vi "Parameter Analyzer.vi"(0 "Function":T3, 1 "Acquisition Mode":T7, 2 "User Integration Time":T9={"Integration Time"=0, "Short Integration Time (s)"=0.0, "Long Integration Time (s)"=0.0, "Wait Time Parameter"=1.0} caption="Sweeping Time Parameters" {"Long Integration Time (s)" scale=0.02..2.0; "Short Integration Time (s)" scale=8e-05..0.00192; "Integration Time" items=["Short", "Long"]; "Wait Time Parameter" format="%.1f"}, 3 "Status Polling Time (ms)":u32=1000, 4 "VISA Session":refnum<visa-resource-name>="GPIB0::27::INSTR", 5 "Comment":string="Test VI", 6 "HP4155C Refnums":T5, 7 "Error in":errorcluster, 8 "SMU 1 - Sweeping":T8={"Start / Offset"=0.0, "Stop / Ratio"=1.0, "Step \n(linear only)"=0.01, "Compliance"=0.1, "Power \nCompliance"=0.0, "Mode"=0, "Function"=0, "Sweep Mode"=FALSE} caption="SMU 1" {"Function" items=["Disabled", "Var 1", "Var 2", "Var 1'", "Constant"]; "Mode" items=["V", "I", "V pulse", "I  pulse", "Common"]; "Power \nCompliance" format="%^.2e"; "Compliance" format="%^.2e"; "Step \n(linear only)" format="%^.4e"; "Stop / Ratio" format="%^.4e"; "Start / Offset" format="%^.4e"}, 9 "SMU1 - Sampling":T12={"Source"=10.0, "Compliance"=1e-05, "Mode"=0, "Function"=FALSE} caption="SMU 1" {"Mode" items=["V", "I", "Common"]; "Compliance" format="%^.2e"; "Source" format="%^.3e"}, 10 "SMU 2 - Sweeping":T8={"Start / Offset"=0.0, "Stop / Ratio"=1.0, "Step \n(linear only)"=0.01, "Compliance"=0.1, "Power \nCompliance"=0.0, "Mode"=0, "Function"=0, "Sweep Mode"=FALSE} caption="SMU 2" {"Function" items=["Disabled", "Var 1", "Var 2", "Var 1'", "Constant"]; "Mode" items=["V", "I", "V pulse", "I  pulse", "Common"]; "Power \nCompliance" format="%^.2e"; "Compliance" format="%^.2e"; "Step \n(linear only)" format="%^.4e"; "Stop / Ratio" format="%^.4e"; "Start / Offset" format="%^.4e"}, 11 "SMU2 - Sampling":T12={"Source"=10.0, "Compliance"=1e-05, "Mode"=0, "Function"=FALSE} caption="SMU 2" {"Mode" items=["V", "I", "Common"]; "Compliance" format="%^.2e"; "Source" format="%^.3e"}, 12 "SMU 3 - Sweeping":T8={"Start / Offset"=0.0, "Stop / Ratio"=1.0, "Step \n(linear only)"=0.01, "Compliance"=0.1, "Power \nCompliance"=0.0, "Mode"=0, "Function"=0, "Sweep Mode"=FALSE} caption="SMU 3" {"Function" items=["Disabled", "Var 1", "Var 2", "Var 1'", "Constant"]; "Mode" items=["V", "I", "V pulse", "I  pulse", "Common"]; "Power \nCompliance" format="%^.2e"; "Compliance" format="%^.2e"; "Step \n(linear only)" format="%^.4e"; "Stop / Ratio" format="%^.4e"; "Start / Offset" format="%^.4e"}, 13 "SMU3 - Sampling":T12={"Source"=10.0, "Compliance"=1e-05, "Mode"=0, "Function"=FALSE} caption="SMU 3" {"Mode" items=["V", "I", "Common"]; "Compliance" format="%^.2e"; "Source" format="%^.3e"}, 14 "SMU 4 - Sweeping":T8={"Start / Offset"=0.0, "Stop / Ratio"=1.0, "Step \n(linear only)"=0.01, "Compliance"=0.1, "Power \nCompliance"=0.0, "Mode"=0, "Function"=0, "Sweep Mode"=FALSE} caption="SMU 4" {"Function" items=["Disabled", "Var 1", "Var 2", "Var 1'", "Constant"]; "Mode" items=["V", "I", "V pulse", "I  pulse", "Common"]; "Power \nCompliance" format="%^.2e"; "Compliance" format="%^.2e"; "Step \n(linear only)" format="%^.4e"; "Stop / Ratio" format="%^.4e"; "Start / Offset" format="%^.4e"}, 15 "SMU4 - Sampling":T12={"Source"=10.0, "Compliance"=1e-05, "Mode"=0, "Function"=FALSE} caption="SMU 4" {"Mode" items=["V", "I", "Common"]; "Compliance" format="%^.2e"; "Source" format="%^.3e"}, 16 "Sweep Spacing":T11 items=["linear", "log 10", "log 25", "log 50"], 17 "Sampling Time Parameters":T13={"Initial Interval (s)"=0.1, "Number of Samples"=60, "Total Sampling Time (s)"=10.0, "Hold Time (s)"=0.0, "Sampling Mode"=0, "Sampling Time"=0} {"Sampling Time" items=["Auto (linear only)", "No Limit", "Set Limit"]; "Sampling Mode" items=["Linear", "Log10", "Log25", "Log50", "Thinned Out"]; "Hold Time (s)" format="%.4f"; "Total Sampling Time (s)" format="%.1f"; "Initial Interval (s)" format="%^.3e"}, 18 "Range":T10 items=["auto", "fixed", "limited"], 19 "Stop Condition":T14={"Enable Delay (s)"=0.0, "Name"="", "Threshold"=0.0, "num. of events"=1, "Event"=0, "Stop Condition Enable"=FALSE} {"Event" items=["Value > Threshold", "Value < Threshold", "| Value | > | Threshold |", "| Value | < | Threshold |"]; "Threshold" format="%^.2e"; "Enable Delay (s)" format="%.1f"}, 20 "Parameter Analyzer Notifiers":T4) -> (22 "Electrical Measurement":T15, 27 "error out":errorcluster)   [LabVIEW 2014]
uses:
  Parameter Analyzer Integration Parameters.ctl
  Electrical Data.ctl
  Parameter Analyzer SMU Sweeping.ctl
  Parameter Analyzer Sweep Spacing.ctl
  Parameter Analyzer Mode Selector.ctl
  Parameter Analyzer Sampling Parameters.ctl
  Parameter Analyzer Stop Sampling Conditions.ctl
  Parameter Analyzer SMU Sampling.ctl
  Parameter Analyzer Refnums.ctl
  Measurements/Plot Data/Electrical Data Plot Refnums.ctl
  Parameter Analyzer Notifiers.ctl
  Parameter Analyzer Functions.ctl
  Parameter Analyzer SMU Range.ctl
  support/Instrument Status.ctl
  support/Instrument Status State.ctl
  <instrlib>/Agilent 415X Series/Agilent 415X Series.lvlib
panel:
  in  "Electrical Measurement":T1(tab)
  out "Current Plot 2":cluster{"Time":dbl[], "SMU4":dbl[]}[](graph)=[{"Time"=[0.0, 0.30000000000000004, 0.6000000000000001, 0.9, 1.2000000000000002, 1.5, 1.8, 2.1, 2.4000000000000004, 2.7, 3.0, 3.3000000000000003, 3.6, 3.9000000000000004, 4.2, 4.5, 4.800000000000001, 5.1000000000000005, 5.4, 5.7, 6.0, 6.300000000000001, 6.6000000000000005, 6.9, 7.2, 7.5, 7.800000000000001, 8.1, 8.4, 8.700000000000001, 9.0, 9.3, 9.600000000000001, 9.9, 10.200000000000001, 10.5, 10.8, 11.100000000000001, 11.4, 11.700000000000001, 12.0, 12.3, 12.600000000000001, 12.9, 13.200000000000001, 13.5, 13.8, 14.100000000000001, 14.4, 14.700000000000001, 15.0, 15.3, 15.600000000000001, 15.9, 16.2, 16.5, 16.8, 17.1, 17.400000000000002, 17.7], "SMU4"=[9.99995e-06, 9.99995e-06, 9.99995e-06, 9.99997e-06, 9.99997e-06, 9.99997e-06, 9.99997e-06, 9.999980000000001e-06, 9.99997e-06, 9.999980000000001e-06, 9.99997e-06, 9.999980000000001e-06, 9.99997e-06, 9.99997e-06, 9.99997e-06, 9.99996e-06, 9.99996e-06, 9.99996e-06, 9.99996e-06, 9.99997e-06, 9.99997e-06, 9.999980000000001e-06, 9.99997e-06, 9.99997e-06, 9.99997e-06, 9.99997e-06, 9.99997e-06, 9.999980000000001e-06, 9.999980000000001e-06, 9.99996e-06, 9.99997e-06, 9.99996e-06, 9.99997e-06, 9.99997e-06, 9.99997e-06, 9.99997e-06, 9.999980000000001e-06, 9.99997e-06, 9.999980000000001e-06, 9.999980000000001e-06, 9.99997e-06, 9.99997e-06, 9.99997e-06, 9.99996e-06, 9.99996e-06, 9.99997e-06, 9.99997e-06, 9.99996e-06, 9.99996e-06, 9.99997e-06, 9.99997e-06, 9.99997e-06, 9.99997e-06, 9.99997e-06, 9.99996e-06, 9.99997e-06, 9.99997e-06, 9.99997e-06, 9.99997e-06, 9.99996e-06]}, {"Time"=[0.0, 0.30000000000000004, 0.6000000000000001, 0.9, 1.2000000000000002, 1.5, 1.8, 2.1, 2.4000000000000004, 2.7, 3.0, 3.3000000000000003, 3.6, 3.9000000000000004, 4.2, 4.5, 4.800000000000001, 5.1000000000000005, 5.4, 5.7, 6.0, 6.300000000000001, 6.6000000000000005, 6.9, 7.2, 7.5, 7.800000000000001, 8.1, 8.4, 8.700000000000001, 9.0, 9.3, 9.600000000000001, 9.9, 10.200000000000001, 10.5, 10.8, 11.100000000000001, 11.4, 11.700000000000001, 12.0, 12.3, 12.600000000000001, 12.9, 13.200000000000001, 13.5, 13.8, 14.100000000000001, 14.4, 14.700000000000001, 15.0, 15.3, 15.600000000000001, 15.9, 16.2, 16.5, 16.8, 17.1, 17.400000000000002, 17.7], "SMU4"=[-1.00004e-05, -1.000039e-05, -1.000039e-05, -1.0000409999999999e-05, -1.000039e-05, -1.000039e-05, -1.00004e-05, -1.000043e-05, -1.000042e-05, -1.0000409999999999e-05, -1.000039e-05, -1.000039e-05, -1.0000409999999999e-05, -1.00004e-05, -1.000038e-05, -1.000038e-05, -1.000039e-05, -1.000037e-05, -1.000038e-05, -1.000039e-05, -1.000039e-05, -1.000039e-05, -1.000039e-05, -1.000039e-05, -1.00004e-05, -1.000037e-05, -1.000038e-05, -1.000039e-05, -1.00004e-05, -1.00004e-05, -1.00004e-05, -1.000037e-05, -1.000037e-05, -1.000037e-05, -1.000036e-05, -1.000039e-05, -1.000038e-05, -1.000037e-05, -1.000036e-05, -1.000037e-05, -1.000038e-05, -1.000037e-05, -1.000038e-05, -1.000036e-05, -1.000037e-05, -1.000037e-05, -1.000037e-05, -1.000039e-05, -1.000038e-05, -1.000036e-05, -1.000037e-05, -1.000039e-05, -1.000036e-05, -1.000037e-05, -1.000038e-05, -1.00004e-05, -1.0000409999999999e-05, -1.000038e-05, -1.000038e-05, -1.00004e-05]}]
  out "Voltage Plot 2":cluster{"Time":dbl[], "SMU4":dbl[]}[](graph)=[{"Time"=[0.0, 0.30000000000000004, 0.6000000000000001, 0.9, 1.2000000000000002, 1.5, 1.8, 2.1, 2.4000000000000004, 2.7, 3.0, 3.3000000000000003, 3.6, 3.9000000000000004, 4.2, 4.5, 4.800000000000001, 5.1000000000000005, 5.4, 5.7, 6.0, 6.300000000000001, 6.6000000000000005, 6.9, 7.2, 7.5, 7.800000000000001, 8.1, 8.4, 8.700000000000001, 9.0, 9.3, 9.600000000000001, 9.9, 10.200000000000001, 10.5, 10.8, 11.100000000000001, 11.4, 11.700000000000001, 12.0, 12.3, 12.600000000000001, 12.9, 13.200000000000001, 13.5, 13.8, 14.100000000000001, 14.4, 14.700000000000001, 15.0, 15.3, 15.600000000000001, 15.9, 16.2, 16.5, 16.8, 17.1, 17.400000000000002, 17.7], "SMU4"=[9.99995e-06, 9.99995e-06, 9.99995e-06, 9.99997e-06, 9.99997e-06, 9.99997e-06, 9.99997e-06, 9.999980000000001e-06, 9.99997e-06, 9.999980000000001e-06, 9.99997e-06, 9.999980000000001e-06, 9.99997e-06, 9.99997e-06, 9.99997e-06, 9.99996e-06, 9.99996e-06, 9.99996e-06, 9.99996e-06, 9.99997e-06, 9.99997e-06, 9.999980000000001e-06, 9.99997e-06, 9.99997e-06, 9.99997e-06, 9.99997e-06, 9.99997e-06, 9.999980000000001e-06, 9.999980000000001e-06, 9.99996e-06, 9.99997e-06, 9.99996e-06, 9.99997e-06, 9.99997e-06, 9.99997e-06, 9.99997e-06, 9.999980000000001e-06, 9.99997e-06, 9.999980000000001e-06, 9.999980000000001e-06, 9.99997e-06, 9.99997e-06, 9.99997e-06, 9.99996e-06, 9.99996e-06, 9.99997e-06, 9.99997e-06, 9.99996e-06, 9.99996e-06, 9.99997e-06, 9.99997e-06, 9.99997e-06, 9.99997e-06, 9.99997e-06, 9.99996e-06, 9.99997e-06, 9.99997e-06, 9.99997e-06, 9.99997e-06, 9.99996e-06]}, {"Time"=[0.0, 0.30000000000000004, 0.6000000000000001, 0.9, 1.2000000000000002, 1.5, 1.8, 2.1, 2.4000000000000004, 2.7, 3.0, 3.3000000000000003, 3.6, 3.9000000000000004, 4.2, 4.5, 4.800000000000001, 5.1000000000000005, 5.4, 5.7, 6.0, 6.300000000000001, 6.6000000000000005, 6.9, 7.2, 7.5, 7.800000000000001, 8.1, 8.4, 8.700000000000001, 9.0, 9.3, 9.600000000000001, 9.9, 10.200000000000001, 10.5, 10.8, 11.100000000000001, 11.4, 11.700000000000001, 12.0, 12.3, 12.600000000000001, 12.9, 13.200000000000001, 13.5, 13.8, 14.100000000000001, 14.4, 14.700000000000001, 15.0, 15.3, 15.600000000000001, 15.9, 16.2, 16.5, 16.8, 17.1, 17.400000000000002, 17.7], "SMU4"=[-1.00004e-05, -1.000039e-05, -1.000039e-05, -1.0000409999999999e-05, -1.000039e-05, -1.000039e-05, -1.00004e-05, -1.000043e-05, -1.000042e-05, -1.0000409999999999e-05, -1.000039e-05, -1.000039e-05, -1.0000409999999999e-05, -1.00004e-05, -1.000038e-05, -1.000038e-05, -1.000039e-05, -1.000037e-05, -1.000038e-05, -1.000039e-05, -1.000039e-05, -1.000039e-05, -1.000039e-05, -1.000039e-05, -1.00004e-05, -1.000037e-05, -1.000038e-05, -1.000039e-05, -1.00004e-05, -1.00004e-05, -1.00004e-05, -1.000037e-05, -1.000037e-05, -1.000037e-05, -1.000036e-05, -1.000039e-05, -1.000038e-05, -1.000037e-05, -1.000036e-05, -1.000037e-05, -1.000038e-05, -1.000037e-05, -1.000038e-05, -1.000036e-05, -1.000037e-05, -1.000037e-05, -1.000037e-05, -1.000039e-05, -1.000038e-05, -1.000036e-05, -1.000037e-05, -1.000039e-05, -1.000036e-05, -1.000037e-05, -1.000038e-05, -1.00004e-05, -1.0000409999999999e-05, -1.000038e-05, -1.000038e-05, -1.00004e-05]}]
  out "Differential Resistance":cluster{"V3":dbl[], "I1":dbl[]}[](graph)
  out "Current Voltage Characteristic":cluster{"V3":dbl[], "I1":dbl[]}[](graph)
  out "Instrument Status":T2
  out "Error Messages":string
  out "Status":T16(ring)=enum."idle"
  out "HP Integration Time":T17={"Short Integration Time"=0.00192, "Medium Integration Time"=0.02, "Long Integration Time"=0.32} caption="Integration Time" {"Long Integration Time" format="%^.2e"; "Medium Integration Time" format="%^.2e"; "Short Integration Time" format="%^.2e"}
  # "LICENSED MATERIALS – PROPERTY OF IBM\nCopyright IBM Corp. 2016,\nALL RIGHTS RESERVED"
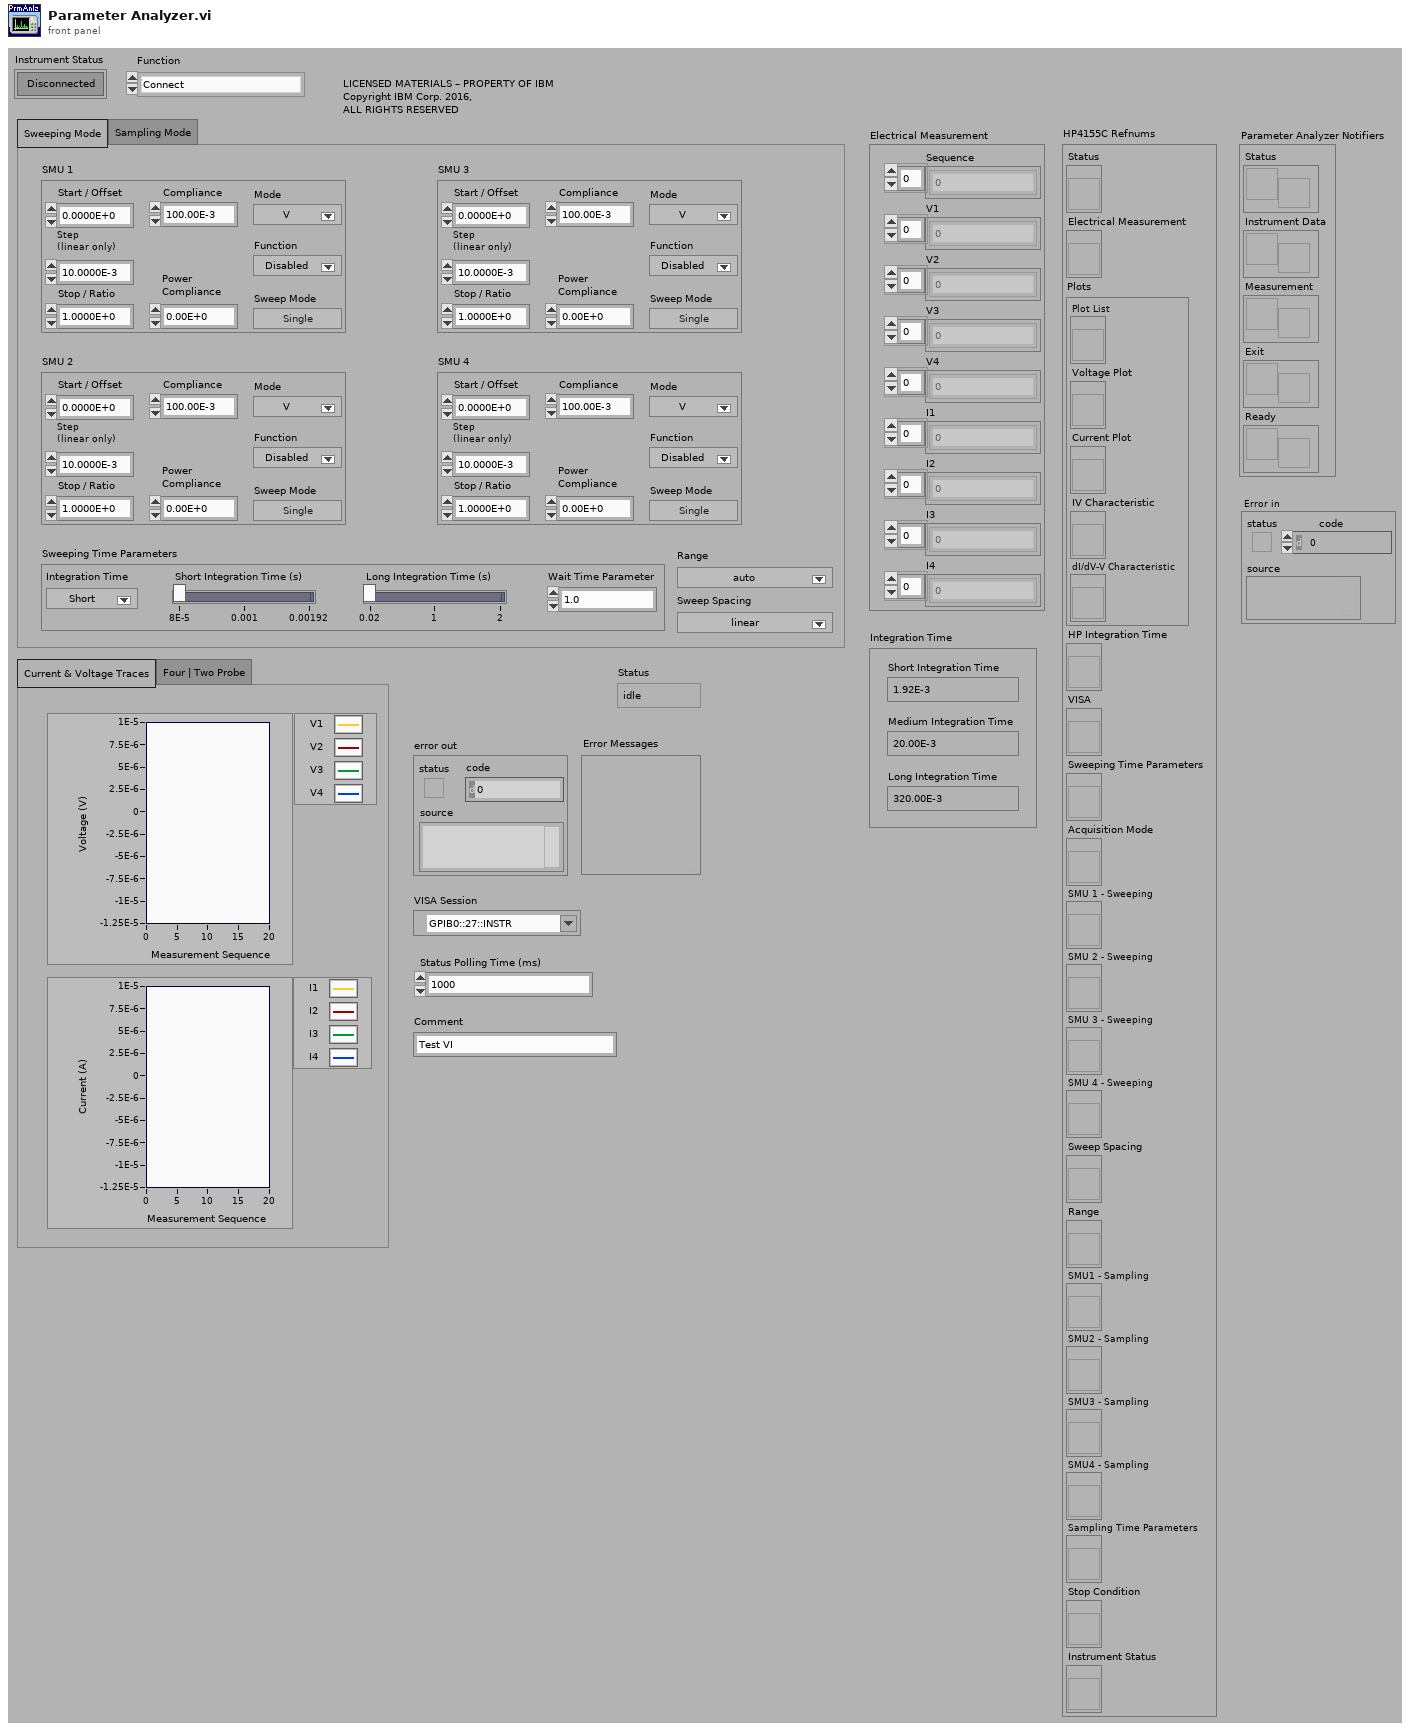
[diagram p1: front panel]
types:
  T1 = enum32{"Current & Voltage Traces", "Four | Two Probe"}
  T2 = typedef "Instrument Status.ctl" = bool
  T3 = typedef "Parameter Analyzer Functions.ctl" = enum16{"Connect", "Configure Sweeping", "Configure Sampling", "Configure Integration Time", "Measure", "Error Check", "Disconnect", "Update Refnums"}
  T4 = typedef "Parameter Analyzer Notifiers.ctl" = cluster{"Status":refnum<notifier>, "Instrument Data":refnum<notifier>, "Measurement":refnum<notifier>, "Exit":refnum<notifier>, "Ready":refnum<notifier>}
  T5 = typedef "Parameter Analyzer Refnums.ctl" = cluster{"Status":refnum<vi>, "Electrical Measurement":refnum<vi>, "Plots":T6, "HP Integration Time":refnum<vi>, "VISA":refnum<vi>, "Sweeping Time Parameters":refnum<vi>, "Acquisition Mode":refnum<vi>, "SMU 1 - Sweeping":refnum<vi>, "SMU 2 - Sweeping":refnum<vi>, "SMU 3 - Sweeping":refnum<vi>, "SMU 4 - Sweeping":refnum<vi>, "Sweep Spacing":refnum<vi>, "Range":refnum<vi>, "SMU1 - Sampling":refnum<vi>, "SMU2 - Sampling":refnum<vi>, "SMU3 - Sampling":refnum<vi>, "SMU4 - Sampling":refnum<vi>, "Sampling Time Parameters":refnum<vi>, "Stop Condition":refnum<vi>, "Instrument Status":refnum<vi>}
  T6 = typedef "Electrical Data Plot Refnums.ctl" = cluster{"Plot List":refnum<vi>, "Voltage Plot":refnum<vi>, "Current Plot":refnum<vi>, "IV Characteristic":refnum<vi>, "dI/dV-V Characteristic":refnum<vi>}
  T7 = typedef "Parameter Analyzer Mode Selector.ctl" = enum32{"Sweeping Mode", "Sampling Mode"}
  T8 = typedef "Parameter Analyzer SMU Sweeping.ctl" = cluster{"Start / Offset":dbl, "Stop / Ratio":dbl, "Step \n(linear only)":dbl, "Compliance":dbl, "Power \nCompliance":dbl, "Mode":u32, "Function":i32, "Sweep Mode":bool}
  T9 = typedef "Parameter Analyzer Integration Parameters.ctl" = cluster{"Integration Time":u32, "Short Integration Time (s)":dbl, "Long Integration Time (s)":dbl, "Wait Time Parameter":dbl}
  T10 = typedef "Parameter Analyzer SMU Range.ctl" = u16
  T11 = typedef "Parameter Analyzer Sweep Spacing.ctl" = u16
  T12 = typedef "Parameter Analyzer SMU Sampling.ctl" = cluster{"Source":dbl, "Compliance":dbl, "Mode":u32, "Function":bool}
  T13 = typedef "Parameter Analyzer Sampling Parameters.ctl" = cluster{"Initial Interval (s)":dbl, "Number of Samples":i32, "Total Sampling Time (s)":dbl, "Hold Time (s)":dbl, "Sampling Mode":i32, "Sampling Time":i32}
  T14 = typedef "Parameter Analyzer Stop Sampling Conditions.ctl" = cluster{"Enable Delay (s)":dbl, "Name":string, "Threshold":dbl, "num. of events":i32, "Event":i32, "Stop Condition Enable":bool}
  T15 = typedef "Electrical Data.ctl" = cluster{"Sequence":dbl[], "V1":dbl[], "V2":dbl[], "V3":dbl[], "V4":dbl[], "I1":dbl[], "I2":dbl[], "I3":dbl[], "I4":dbl[]}
  T16 = enum16{"unknown", "idle", "standby", "measurement", "stress force"}
  T17 = cluster{"Short Integration Time":dbl, "Medium Integration Time":dbl, "Long Integration Time":dbl}
  T18 = typedef "Instrument Status State.ctl" = enum16{"Unknown", "Idle", "Standby", "Configuring", "Measuring", "Moving", "Disconnected"}
  T19 = cluster{"unit (VMU1:0)":u16, "range (fixed:1)":u16, "SMU I range\n(1 nA:2)":u16, "SMU V range\n(2 V:0)":u16, "VMU range\n(2 V:1)":u16}[]
  T20 = cluster{"unit (VMU1:0)":u16, "range (fixed:1)":u16, "SMU I range\n(1 nA:2)":u16, "SMU V range\n(2 V:0)":u16, "VMU range\n(2 V:1)":u16}
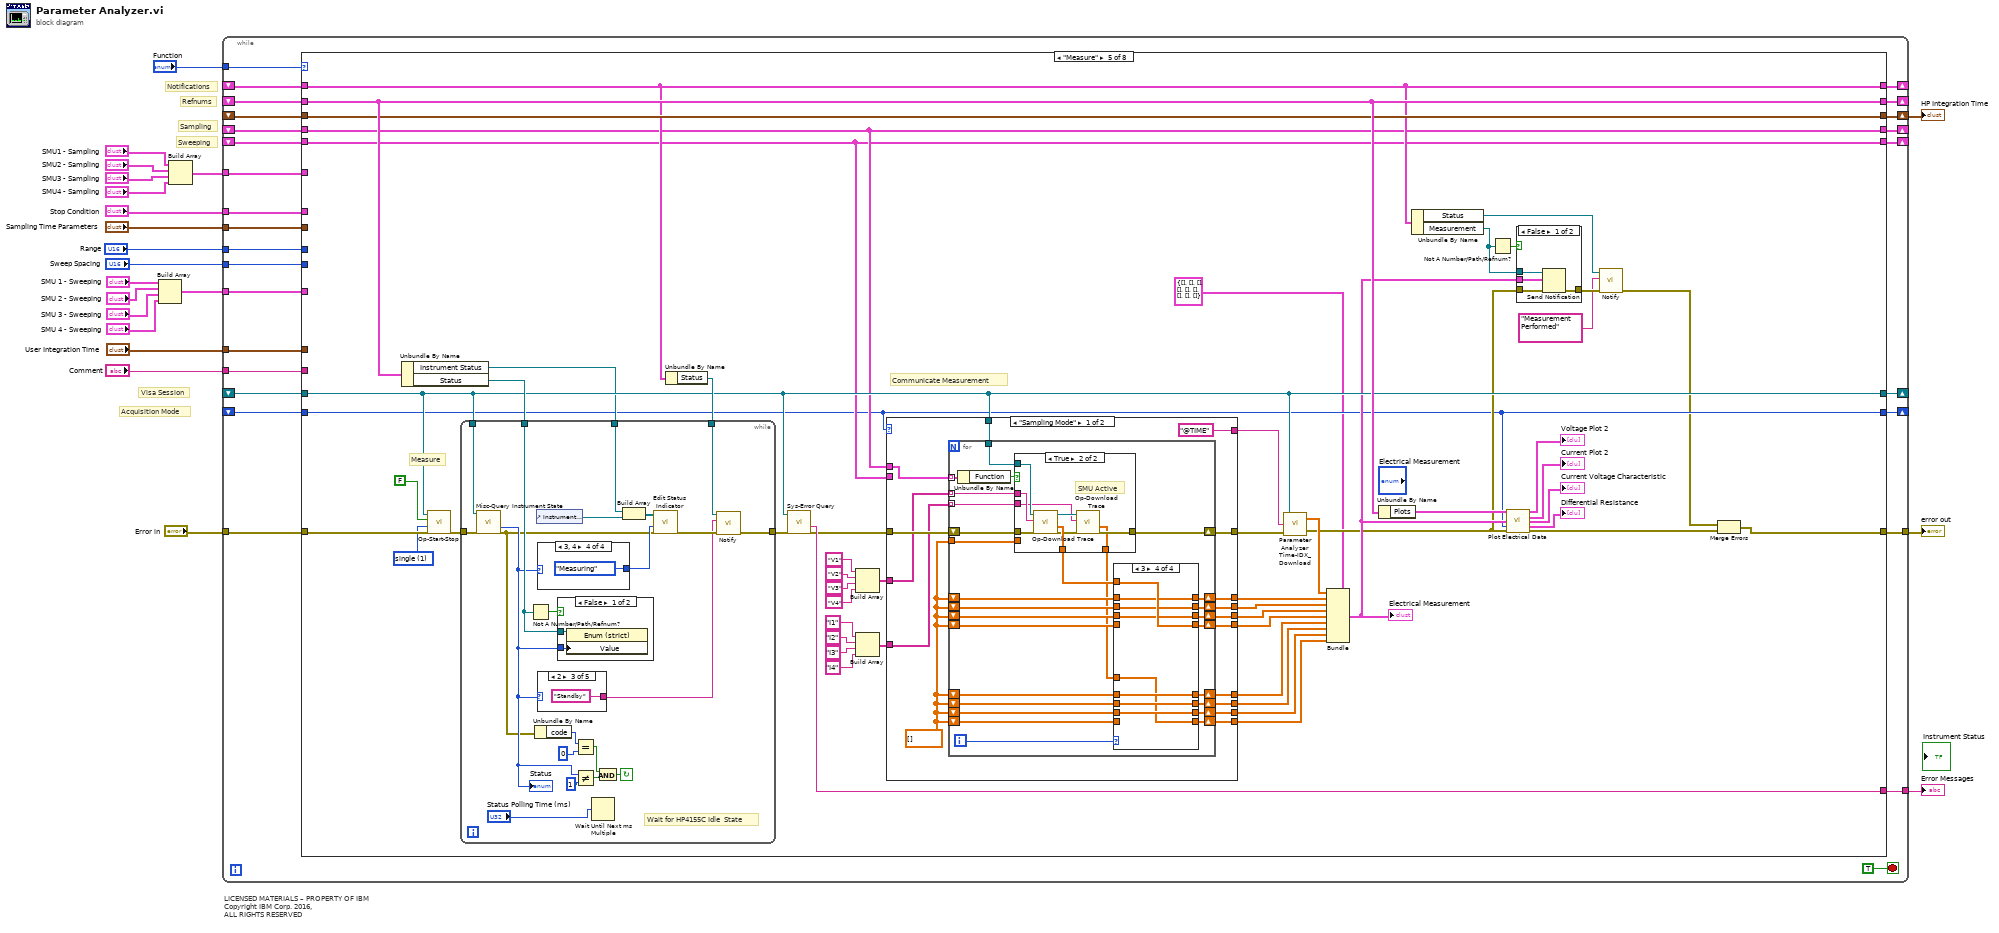
[diagram p0: block diagram]
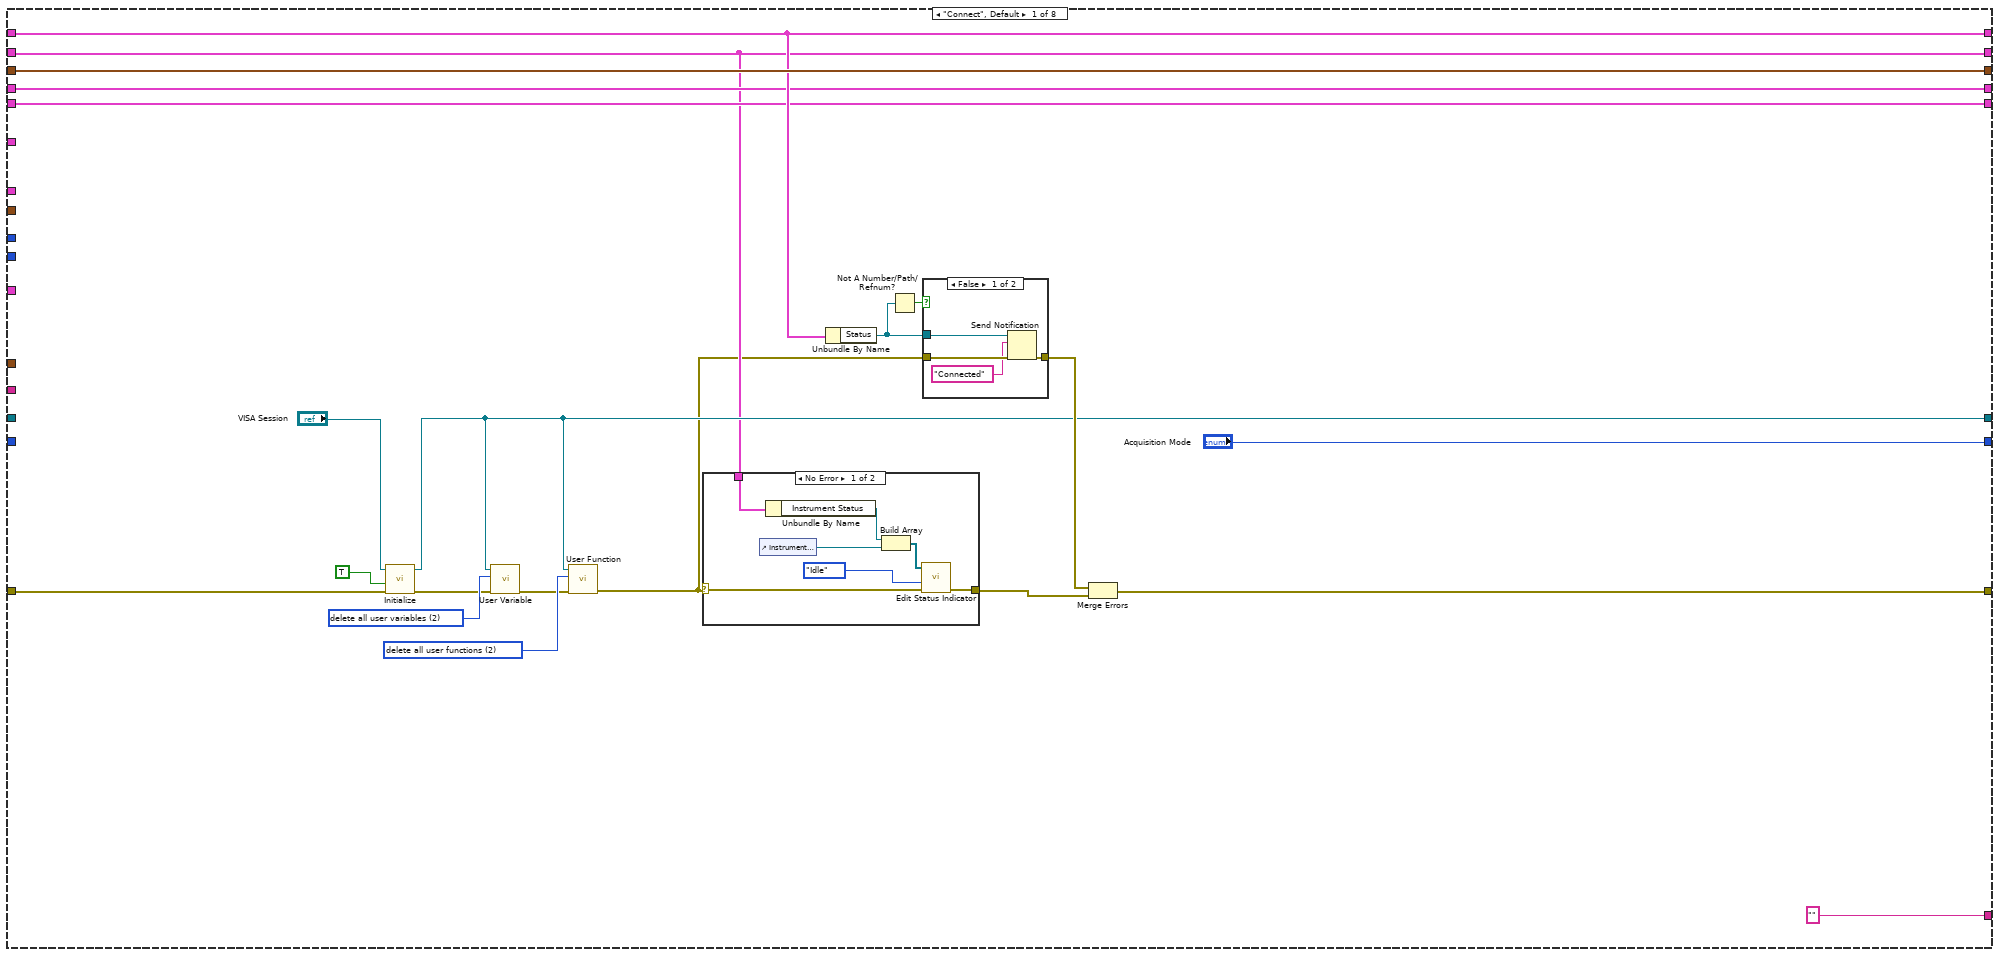
[diagram p2: hidden frame]
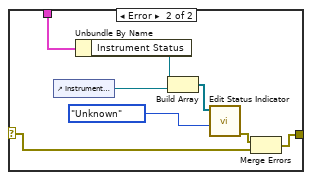
[diagram p3: hidden frame]
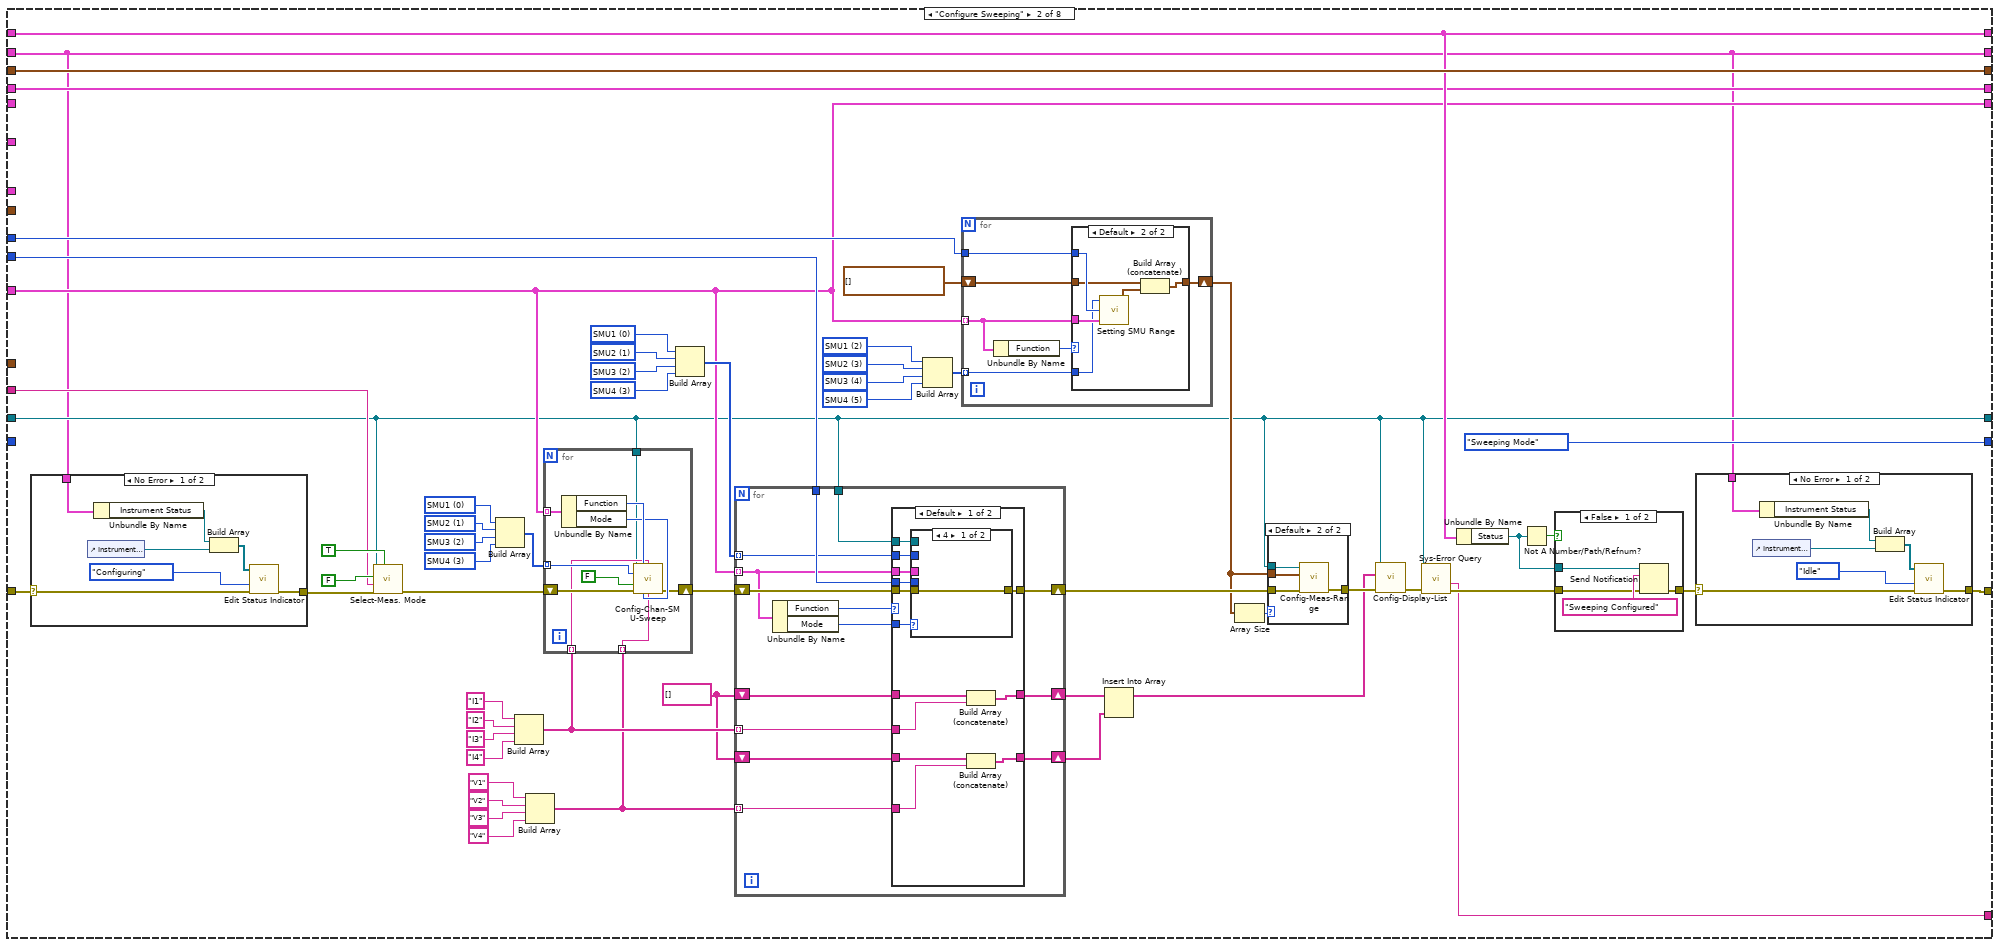
[diagram p5: hidden frame]
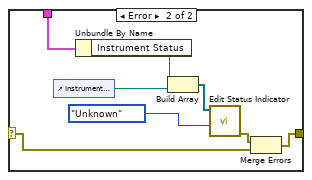
[diagram p6: hidden frame]
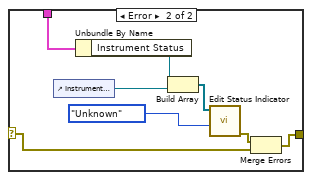
[diagram p7: hidden frame]
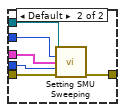
[diagram p9: hidden frame]
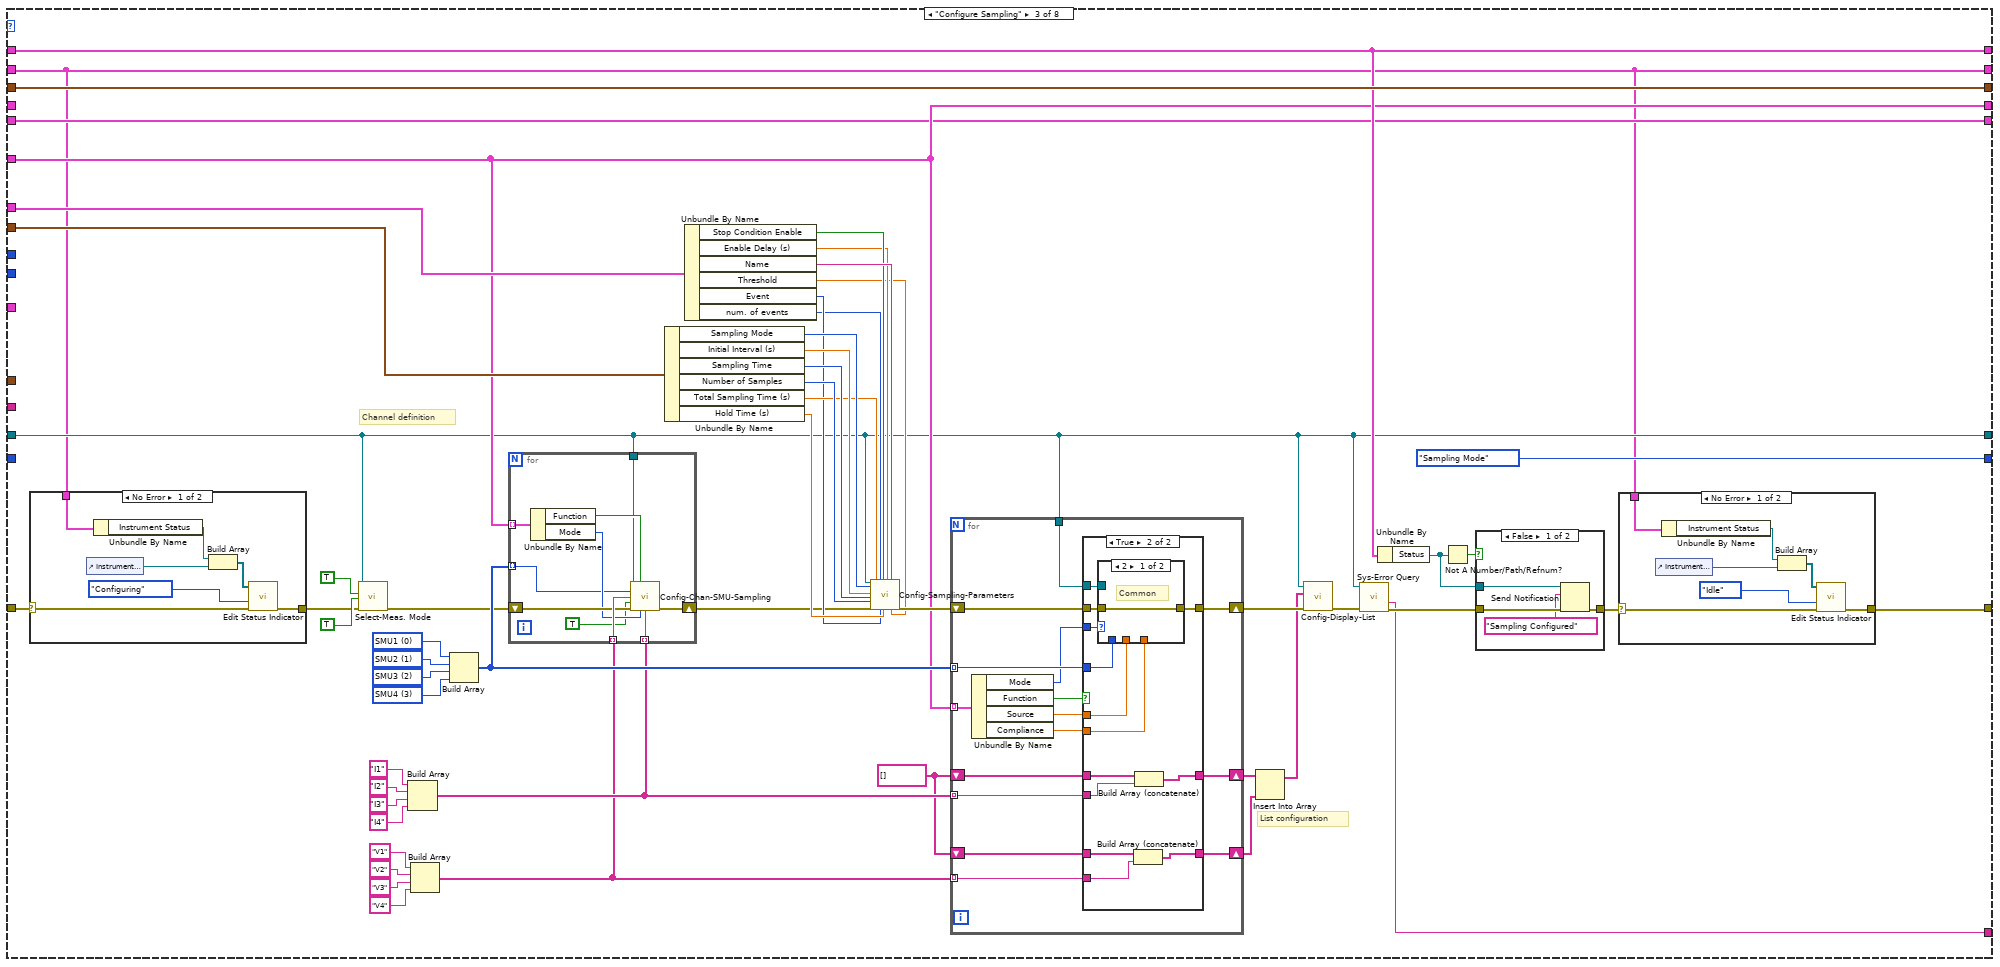
[diagram p13: hidden frame]
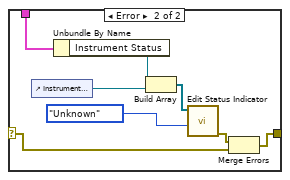
[diagram p14: hidden frame]
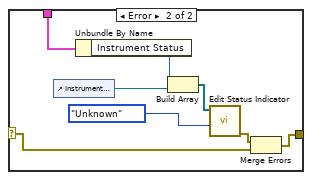
[diagram p15: hidden frame]
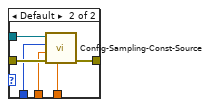
[diagram p17: hidden frame]
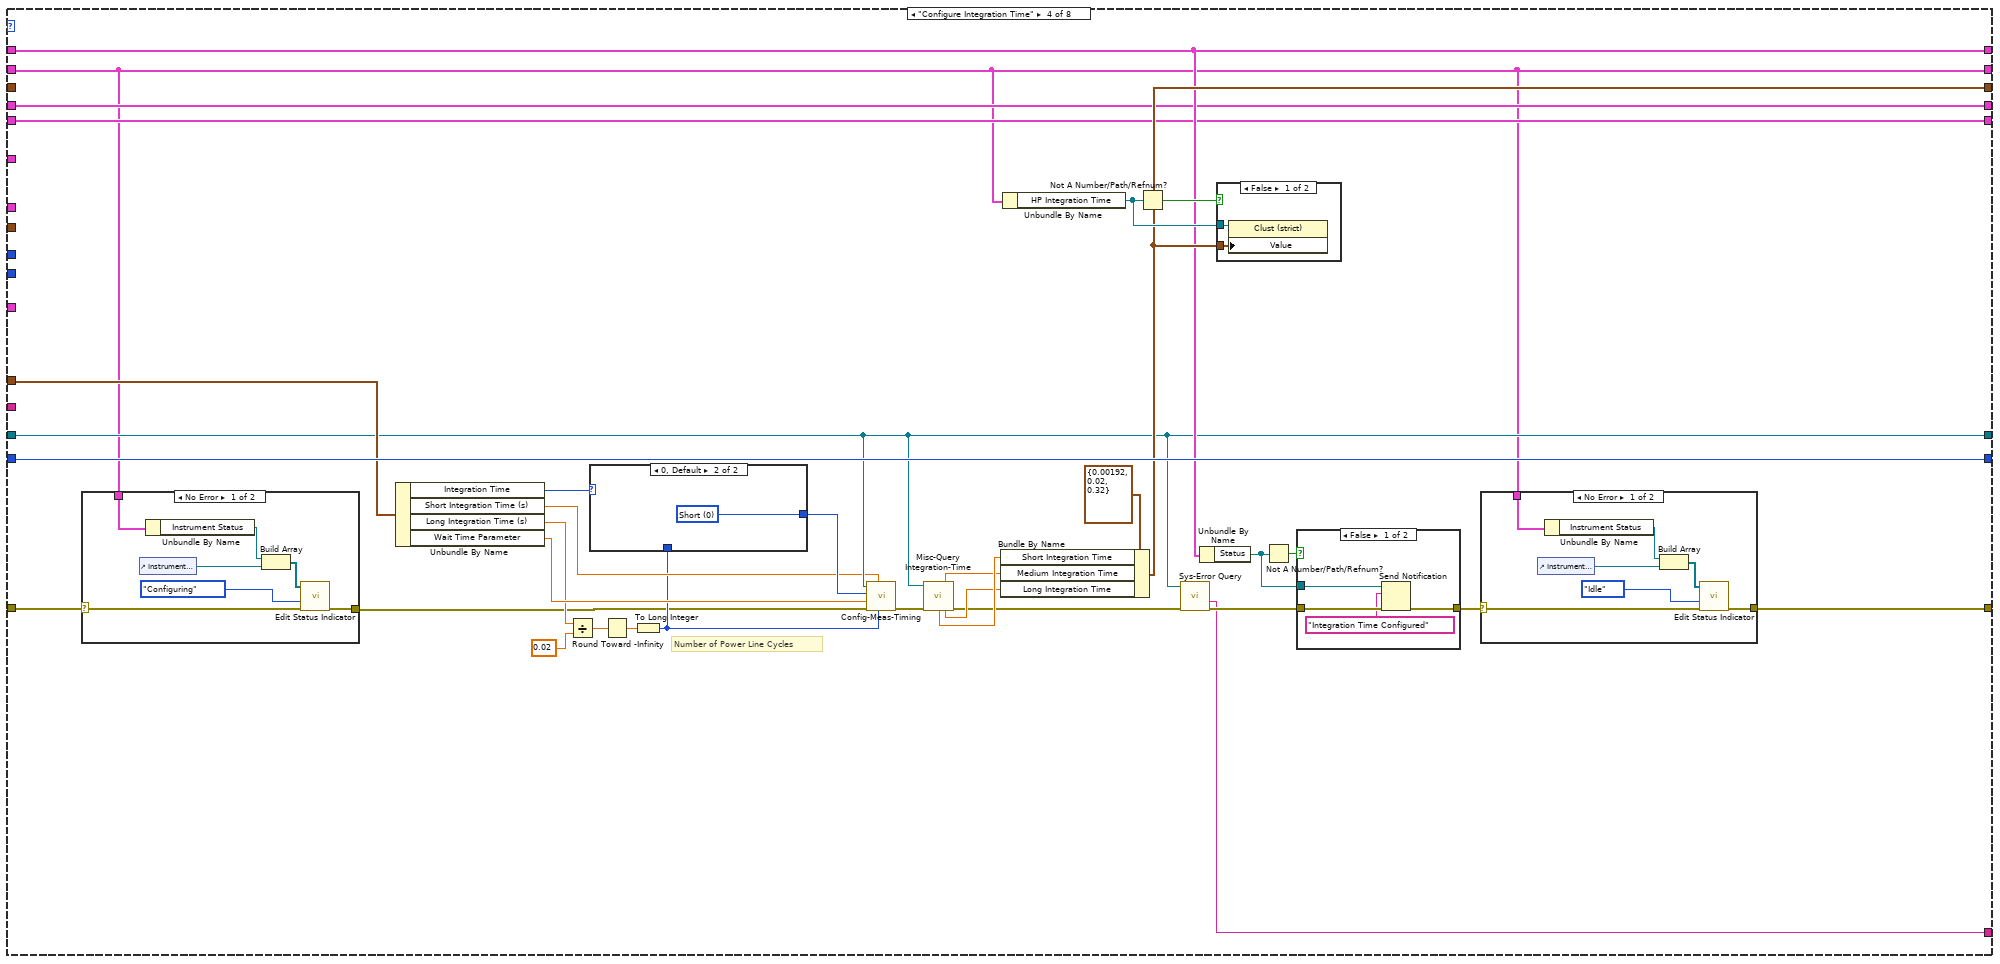
[diagram p19: hidden frame]
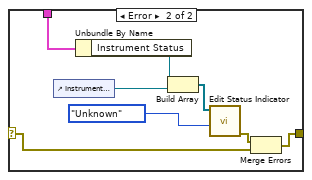
[diagram p20: hidden frame]
diagram:
  # "LICENSED MATERIALS – PROPERTY OF IBM\nCopyright IBM Corp. 2016,\nALL RIGHTS RESERVED"
  # "Sweeping"
  # "Sampling"
  # "Notifications"
  # "Refnums"
  # "Acquisition Mode"
  # "Visa Session"
  n1 = Build Array("SMU 1 - Sweeping", "SMU 2 - Sweeping", "SMU 3 - Sweeping", "SMU 4 - Sweeping") -> (w1:T8[])
  n2 = Build Array("SMU1 - Sampling", "SMU2 - Sampling", "SMU3 - Sampling", "SMU4 - Sampling") -> (w6:T12[])
  n3 = while {
    tunnel: "Function" -> [w47]
    tunnel: [w46] -> w11
    tunnel: "Error in" -> [w45]
    shift-right: [w44] -> _
    shift-left: _ -> [w43]
    tunnel: "Comment" -> [w42]
    shift-right: [w41] -> _
    shift-left: _ -> [w40]
    shift-right: [w39] -> _
    shift-left: _ -> [w38]
    shift-right: [w36] -> w18
    shift-left: _ -> [w35]
    shift-right: [w34] -> _
    shift-left: _ -> [w33]
    tunnel: "User Integration Time" -> [w32]
    tunnel: "Stop Condition" -> [w31]
    tunnel: "Sampling Time Parameters" -> [w30]
    tunnel: [w37] -> w19
    tunnel: "Range" -> [w29]
    tunnel: "Sweep Spacing" -> [w28]
    shift-right: [w23] -> _
    shift-left: _ -> [w22]
    tunnel: w6 -> [w27]
    tunnel: w1 -> [w26]
    shift-right: [w24] -> _
    shift-left: _ -> [w25]
    stop <- TRUE stop-if-true
    n4 = case shown="\"Measure\"" w47 {
      tunnel: [w51 w90 w247 w385 w467 w731 w734 w767] -> w46
      tunnel: w45 -> [w69 w94 w251 w389 w510 w730 w746 w768]
      tunnel: [w55 w103 w258 w402 w491 w729 w745 w778] -> w44
      tunnel: w43 -> [_ w103 w258 w402 w491 w729 w745 w778]
      tunnel: w42 -> [_ w143 _ _ _ _ _ _]
      tunnel: ["Acquisition Mode" enum32{"Sweeping Mode", "Sampling Mode"}."Sweeping Mode" ("Acquisition Mode 2") enum32{"Sweeping Mode", "Sampling Mode"}."Sampling Mode" ("Acquisition Mode 2") w417 w465 w728 w744 w777] -> w41
      tunnel: w40 -> [_ _ _ w417 w465 w728 w744 w777]
      tunnel: [w52 w92 w248 w386 w509 w727 w735 "HP4155C Refnums"] -> w39
      tunnel: w38 -> [w52 w92 w248 w386 w509 w727 w735 _]
      tunnel: ["" ("messages") w137 w290 w401 w502 w726 "" ("messages") "" ("messages")] -> w37
      tunnel: [w66 w142 w297 w409 w507 w725 w743 w775] -> w36
      tunnel: w35 -> [w66 w142 w297 _ w507 w725 w743 w775]
      tunnel: [w64 w141 w294 w406 w501 w724 w739 "Parameter Analyzer Notifiers"] -> w34
      tunnel: w33 -> [w64 w141 w294 w406 w501 w724 w739 _]
      tunnel: w32 -> [_ _ _ w405 _ _ _ _]
      tunnel: w31 -> [_ _ w293 _ _ _ _ _]
      tunnel: w30 -> [_ _ w292 _ _ _ _ _]
      tunnel: w29 -> [_ w120 _ _ _ _ _ _]
      tunnel: w28 -> [_ w118 _ _ _ _ _ _]
      tunnel: w27 -> [_ _ w263 _ _ _ _ _]
      tunnel: w26 -> [_ w107 _ _ _ _ _ _]
      tunnel: w25 -> [w56 _ w262 w390 w476 w722 w736 w771]
      tunnel: [w56 w107 w262 w390 w476 w722 w736 w771] -> w24
      tunnel: [w57 w106 w263 w391 w477 w723 w737 w772] -> w23
      tunnel: w22 -> [w57 w106 _ w391 w477 w723 w737 w772]
      frame "Connect", Default {
        w60 = u32 2 items=["define new function  ", "delete user function by name  ", "delete all user functions  ", "list current user functions  "] ("operation 2")
        w61 = u32 2 items=["define new variable  ", "delete variable by name  ", "delete all user variables  ", "resize user variable by name  ", "list all user variables  "] ("operation")
        n5 = call <instrlib>:"Initialize.vi"("error in (no error)"=w69, "reset"=TRUE, "VISA resource name"="VISA Session") -> ("error out"=w58:errorcluster, "VISA resource name out"=w55:refnum<visa-resource-name>)  [unwired: 2 in, 5 out]
        n6 = call <instrlib>:"User Variable.vi"("error in (no error)"=w58, "operation"=w61, "VISA session"=w55) -> ("error out"=w59:errorcluster)  [unwired: 3 in, 5 out]
        n7 = call <instrlib>:"User Function.vi"("error in (no error)"=w59, "operation"=w60, "VISA session"=w55) -> ("error out"=w49:errorcluster)  [unwired: 3 in, 5 out]
        n8 = case shown="No Error" w49 {
          selector: w49 -> [w75 w79]
          tunnel: [w74 w78] -> w50
          tunnel: w52 -> [w70 w80]
          frame No Error {
            n9 = control-ref of="Instrument Status"() -> (w73:refnum<vi>)
            n10 = Unbundle By Name(w70) -> ("Instrument Status"=w71:refnum<vi>)
            n11 = Build Array(w71, w73) -> (w72:refnum<vi>[])
            n12 = call "Edit Status Indicator.vi"("error in (no error)"=w75, "State"=Instrument_Status_State."Idle", "Instrument Status Refnum"=w72) -> ("error out"=w74:errorcluster)  [unwired: 1 in, 7 out]
          }
          frame Error {
            n13 = control-ref of="Instrument Status"() -> (w83:refnum<vi>)
            n14 = Unbundle By Name(w80) -> ("Instrument Status"=w81:refnum<vi>)
            n15 = Build Array(w81, w83) -> (w82:refnum<vi>[])
            n16 = call "Edit Status Indicator.vi"("State"=Instrument_Status_State."Unknown", "Instrument Status Refnum"=w82) -> ("error out"=w77:errorcluster)  [unwired: 2 in, 7 out]
            n17 = Merge Errors(w77, w79) -> (w78:errorcluster)
          }
        }
        n18 = Unbundle By Name(w64) -> ("Status"=w62:refnum<notifier>)
        n19 = Not A Number/Path/Refnum?(number/path/refnum=w62) -> (NaN/Path/Refnum?=w63:bool)
        n20 = case shown="False" w63 {
          tunnel: w49 -> [w88 w89]
          tunnel: [w87 w89] -> w65
          tunnel: w62 -> [w86 _]
          frame False {
            n21 = Send Notification(notification="Connected", notifier=w86, error in (no error)=w88) -> (error out=w87:errorcluster)  [unwired: 1 out]
          }
          frame True {
          }
        }
        n22 = Merge Errors(w65, w50) -> (w51:errorcluster)
      }
      frame "Configure Sweeping" {
        w98 = string[] []
        w109 = u16 5 items=["VMU1", "VMU2", "SMU1", "SMU2", "SMU3", "SMU4", "SMU5", "SMU6"] ("unit (VMU1:0)")
        w110 = u16 4 items=["VMU1", "VMU2", "SMU1", "SMU2", "SMU3", "SMU4", "SMU5", "SMU6"] ("unit (VMU1:0)")
        w111 = u16 3 items=["VMU1", "VMU2", "SMU1", "SMU2", "SMU3", "SMU4", "SMU5", "SMU6"] ("unit (VMU1:0)")
        w112 = u16 2 items=["VMU1", "VMU2", "SMU1", "SMU2", "SMU3", "SMU4", "SMU5", "SMU6"] ("unit (VMU1:0)")
        w136 = u16 3 items=["SMU 1", "SMU2", "SMU3", "SMU4", "SMU5", "SMU6", "VSU1", "VSU2"] ("Unit To Setup")
        w135 = u16 2 items=["SMU 1", "SMU2", "SMU3", "SMU4", "SMU5", "SMU6", "VSU1", "VSU2"] ("Unit To Setup")
        w134 = u16 1 items=["SMU 1", "SMU2", "SMU3", "SMU4", "SMU5", "SMU6", "VSU1", "VSU2"] ("Unit To Setup")
        w133 = u16 0 items=["SMU1", "SMU2", "SMU3", "SMU4", "SMU5", "SMU6", "VSU1", "VSU2"] ("Unit To Setup")
        w132 = 3 items=["SMU1  ", "SMU2  ", "SMU3  ", "SMU4  ", "SMU5  ", "SMU6  "] ("unit to configure")
        w131 = 2 items=["SMU1  ", "SMU2  ", "SMU3  ", "SMU4  ", "SMU5  ", "SMU6  "] ("unit to configure")
        w130 = 1 items=["SMU1  ", "SMU2  ", "SMU3  ", "SMU4  ", "SMU5  ", "SMU6  "] ("unit to configure")
        w129 = 0 items=["SMU1  ", "SMU2  ", "SMU3  ", "SMU4  ", "SMU5  ", "SMU6  "] ("unit to configure")
        n23 = case shown="No Error" w94 {
          selector: w94 -> [w167 w171]
          tunnel: [w166 w170] -> w93
          tunnel: w92 -> [w162 w172]
          frame No Error {
            n24 = control-ref of="Instrument Status"() -> (w165:refnum<vi>)
            n25 = Unbundle By Name(w162) -> ("Instrument Status"=w163:refnum<vi>)
            n26 = Build Array(w163, w165) -> (w164:refnum<vi>[])
            n27 = call "Edit Status Indicator.vi"("error in (no error)"=w167, "State"=Instrument_Status_State."Configuring", "Instrument Status Refnum"=w164) -> ("error out"=w166:errorcluster)  [unwired: 1 in, 7 out]
          }
          frame Error {
            n28 = control-ref of="Instrument Status"() -> (w175:refnum<vi>)
            n29 = Unbundle By Name(w172) -> ("Instrument Status"=w173:refnum<vi>)
            n30 = Build Array(w173, w175) -> (w174:refnum<vi>[])
            n31 = call "Edit Status Indicator.vi"("State"=Instrument_Status_State."Unknown", "Instrument Status Refnum"=w174) -> ("error out"=w169:errorcluster)  [unwired: 2 in, 7 out]
            n32 = Merge Errors(w169, w171) -> (w170:errorcluster)
          }
        }
        n33 = call <instrlib>:"Select-Meas. Mode.vi"("clear all channels"=TRUE, "error in (no error)"=w93, "comment (\"Setting_1\") (max 58 chars)"=w143, "measurement mode"=FALSE, "VISA resource name"=w103) -> ("error out"=w102:errorcluster)  [unwired: 6 out]
        n34 = Build Array(w129, w130, w131, w132) -> (w101:i32[])
        n35 = Build Array("I1" ("I name (max 6 chars)"), "I2" ("I name (max 6 chars)"), "I3" ("I name (max 6 chars)"), "I4" ("I name (max 6 chars)")) -> (w100:string[])
        n36 = Build Array("V1" ("V name (max 6 chars)"), "V2" ("V name (max 6 chars)"), "V3" ("V name (max 6 chars)"), "V4" ("V name (max 6 chars)")) -> (w99:string[])
        n37 = for {
          tunnel: w101 -> [w227] mode=indexing
          shift-right: [w220] -> w119
          shift-left: w102 -> [w224]
          tunnel: w100 -> [w223] mode=indexing
          tunnel: w99 -> [w222] mode=indexing
          tunnel: w107 -> [w221] mode=indexing
          tunnel: w103 -> [w219]
          n38 = Unbundle By Name(w221) -> ("Function"=w226:i32, "Mode"=w225:u32)
          n39 = call <instrlib>:"Config-Chan-SMU-Sweep.vi"("VISA session"=w219, "function"=w226, "I name (max 6 chars)"=w223, "unit to configure"=w227, "standby"=FALSE, "error in (no error)"=w224, "mode"=w225, "V name (max 6 chars)"=w222) -> ("error out"=w220:errorcluster)  [unwired: 1 in, 6 out]
        }
        n40 = Build Array(w133, w134, w135, w136) -> (w117:u16[])
        n41 = for {
          shift-right: [w195] -> w116
          shift-left: w119 -> [w194]
          tunnel: w118 -> [w193]
          tunnel: w107 -> [w189] mode=indexing
          tunnel: w117 -> [w192] mode=indexing
          tunnel: w103 -> [w191]
          tunnel: w100 -> [w184] mode=indexing
          tunnel: w99 -> [w182] mode=indexing
          shift-right: [w183] -> w97
          shift-left: w98 -> [w187]
          shift-right: [w185] -> w96
          shift-left: w98 -> [w186]
          n42 = Unbundle By Name(w189) -> ("Function"=w190:i32, "Mode"=w188:u32)
          n43 = case shown="Default" w190 {
            tunnel: [w208 w218] -> w195
            tunnel: w194 -> [w207 w218]
            tunnel: w193 -> [w206 _]
            tunnel: w189 -> [w205 _]
            tunnel: w192 -> [w204 _]
            tunnel: w191 -> [w203 _]
            tunnel: w188 -> [w202 _]
            tunnel: w187 -> [w201 w216]
            tunnel: [w200 w216] -> w183
            tunnel: w186 -> [w198 w217]
            tunnel: [w197 w217] -> w185
            tunnel: w184 -> [w199 _]
            tunnel: w182 -> [w196 _]
            frame Default {
              n44 = case shown="4" w202 {
                tunnel: [w209 w215] -> w208
                tunnel: w207 -> [w209 w214]
                tunnel: w206 -> [_ w213]
                tunnel: w205 -> [_ w212]
                tunnel: w204 -> [_ w211]
                tunnel: w203 -> [_ w210]
                frame 4 {
                }
                frame Default {
                  n45 = call "Setting SMU Sweeping.vi"("VISA session"=w210, "Unit To Setup"=w211, "SMU - Sweeping"=w212, "Sweep spacing"=w213, "Error in"=w214) -> ("Error out"=w215:errorcluster)  [unwired: 8 in, 2 out]
                }
              }
              n46 = Build Array (concatenate)(w201, w199) -> (w200:string[])
              n47 = Build Array (concatenate)(w198, w196) -> (w197:string[])
            }
            frame 0 {
              # "SMU Inactive: Don't \nadd it to the list"
            }
          }
        }
        n48 = Build Array(w112, w111, w110, w109) -> (w108:u16[])
        n49 = for {
          tunnel: w107 -> [w231] mode=indexing
          tunnel: w120 -> [w232]
          shift-right: [w233] -> w114
          shift-left: T19 [] ("Array") -> [w234]
          tunnel: w108 -> [w229] mode=indexing
          n50 = Unbundle By Name(w231) -> ("Function"=w230:i32)
          n51 = case shown="Default" w230 {
            tunnel: w234 -> [w235 w238]
            tunnel: [w235 w237] -> w233
            tunnel: w232 -> [_ w241]
            tunnel: w231 -> [_ w240]
            tunnel: w229 -> [_ w239]
            frame 0 {
            }
            frame Default {
              n52 = call "Setting SMU Range.vi"("SMU - Sweeping"=w240, "Range"=w241, "unit (VMU1:0)"=w239) -> ("output cluster"=w236:T20)
              n53 = Build Array (concatenate)(w238, w236) -> (w237:T19)
            }
          }
        }
        n54 = Insert Into Array(array=w97, new element=w96) -> (w95:string[])  [unwired: 1 in]
        n55 = Array Size(array=w114) -> (size(s)=w113:i32)
        n56 = case shown="Default" w113 {
          tunnel: [w177 w181] -> w105
          tunnel: w114 -> [_ w180]
          tunnel: w116 -> [w177 w179]
          tunnel: w103 -> [_ w178]
          frame 0 {
          }
          frame Default {
            n57 = call <instrlib>:"Config-Meas-Range.vi"("error in (no error)"=w179, "measurement range"=w180, "VISA session"=w178) -> ("error out"=w181:errorcluster)  [unwired: 1 in, 7 out]
          }
        }
        n58 = call <instrlib>:"Config-Display-List.vi"("error in (no error)"=w105, "list (max 8 elements)"=w95, "VISA session"=w103) -> ("error out"=w104:errorcluster)  [unwired: 1 in, 7 out]
        n59 = call <instrlib>:"Sys-Error Query.vi"("error in (no error)"=w104, "VISA session"=w103) -> ("error out"=w138:errorcluster, "messages"=w137:string)  [unwired: 1 in, 7 out]
        n60 = Unbundle By Name(w141) -> ("Status"=w140:refnum<notifier>)
        n61 = Not A Number/Path/Refnum?(number/path/refnum=w140) -> (NaN/Path/Refnum?=w139:bool)
        n62 = case shown="False" w139 {
          tunnel: [w245 w246] -> w91
          tunnel: w140 -> [w244 _]
          tunnel: w138 -> [w242 w246]
          frame False {
            n63 = Send Notification(notification="Sweeping Configured", notifier=w244, error in (no error)=w242) -> (error out=w245:errorcluster)  [unwired: 1 out]
          }
          frame True {
          }
        }
        n64 = case shown="No Error" w91 {
          selector: w91 -> [w152 w156]
          tunnel: [w151 w155] -> w90
          tunnel: w92 -> [w147 w157]
          frame No Error {
            n65 = control-ref of="Instrument Status"() -> (w150:refnum<vi>)
            n66 = Unbundle By Name(w147) -> ("Instrument Status"=w148:refnum<vi>)
            n67 = Build Array(w148, w150) -> (w149:refnum<vi>[])
            n68 = call "Edit Status Indicator.vi"("error in (no error)"=w152, "State"=Instrument_Status_State."Idle", "Instrument Status Refnum"=w149) -> ("error out"=w151:errorcluster)  [unwired: 1 in, 7 out]
          }
          frame Error {
            n69 = control-ref of="Instrument Status"() -> (w160:refnum<vi>)
            n70 = Unbundle By Name(w157) -> ("Instrument Status"=w158:refnum<vi>)
            n71 = Build Array(w158, w160) -> (w159:refnum<vi>[])
            n72 = call "Edit Status Indicator.vi"("State"=Instrument_Status_State."Unknown", "Instrument Status Refnum"=w159) -> ("error out"=w154:errorcluster)  [unwired: 2 in, 7 out]
            n73 = Merge Errors(w154, w156) -> (w155:errorcluster)
          }
        }
      }
      frame "Configure Sampling" {
        w255 = string[] []
        w276 = u32 3 items=["SMU1  ", "SMU2  ", "SMU3  ", "SMU4  ", "SMU5  ", "SMU6  "] ("unit to configure")
        w274 = u32 2 items=["SMU1  ", "SMU2  ", "SMU3  ", "SMU4  ", "SMU5  ", "SMU6  "] ("unit to configure")
        w275 = u32 1 items=["SMU1  ", "SMU2  ", "SMU3  ", "SMU4  ", "SMU5  ", "SMU6  "] ("unit to configure")
        w277 = u32 0 items=["SMU1  ", "SMU2  ", "SMU3  ", "SMU4  ", "SMU5  ", "SMU6  "] ("unit to configure")
        # "List configuration"
        # "Channel definition"
        n74 = case shown="No Error" w251 {
          selector: w251 -> [w322 w326]
          tunnel: [w321 w325] -> w250
          tunnel: w248 -> [w317 w327]
          frame No Error {
            n75 = control-ref of="Instrument Status"() -> (w320:refnum<vi>)
            n76 = Unbundle By Name(w317) -> ("Instrument Status"=w318:refnum<vi>)
            n77 = Build Array(w318, w320) -> (w319:refnum<vi>[])
            n78 = call "Edit Status Indicator.vi"("error in (no error)"=w322, "State"=Instrument_Status_State."Configuring", "Instrument Status Refnum"=w319) -> ("error out"=w321:errorcluster)  [unwired: 1 in, 7 out]
          }
          frame Error {
            n79 = control-ref of="Instrument Status"() -> (w330:refnum<vi>)
            n80 = Unbundle By Name(w327) -> ("Instrument Status"=w328:refnum<vi>)
            n81 = Build Array(w328, w330) -> (w329:refnum<vi>[])
            n82 = call "Edit Status Indicator.vi"("State"=Instrument_Status_State."Unknown", "Instrument Status Refnum"=w329) -> ("error out"=w324:errorcluster)  [unwired: 2 in, 7 out]
            n83 = Merge Errors(w324, w326) -> (w325:errorcluster)
          }
        }
        n84 = call <instrlib>:"Select-Meas. Mode.vi"("clear all channels"=TRUE, "error in (no error)"=w250, "measurement mode"=TRUE, "VISA resource name"=w258) -> ("error out"=w261:errorcluster)  [unwired: 1 in, 6 out]
        n85 = Build Array("I1" ("I name (max 6 chars)"), "I2" ("I name (max 6 chars)"), "I3" ("I name (max 6 chars)"), "I4" ("I name (max 6 chars)")) -> (w257:string[])
        n86 = Build Array("V1" ("V name (max 6 chars)"), "V2" ("V name (max 6 chars)"), "V3" ("V name (max 6 chars)"), "V4" ("V name (max 6 chars)")) -> (w256:string[])
        n87 = Build Array(w277, w275, w274, w276) -> (w264:u32[])
        n88 = for {
          tunnel: w257 -> [w379] mode=indexing
          tunnel: w256 -> [w378] mode=indexing
          shift-right: [w376] -> w265
          shift-left: w261 -> [w377]
          tunnel: w264 -> [w373] mode=indexing
          tunnel: w263 -> [w371] mode=indexing
          tunnel: w258 -> [w370]
          n89 = Unbundle By Name(w371) -> ("Function"=w374:bool, "Mode"=w375:u32)
          n90 = call <instrlib>:"Config-Chan-SMU-Sampling.vi"("VISA resource name in"=w370, "function"=w374, "unit to configure"=w373, "V name (max 6 chars)"=w378, "standby"=TRUE, "error in (no error)"=w377, "mode"=w375, "I name (max 6 chars)"=w379) -> ("error out"=w376:errorcluster)  [unwired: 1 in, 6 out]
        }
        n91 = Unbundle By Name(w292) -> ("Sampling Mode"=w289:i32, "Initial Interval (s)"=w288:dbl, "Sampling Time"=w287:i32, "Number of Samples"=w286:i32, "Total Sampling Time (s)"=w284:dbl, "Hold Time (s)"=w283:dbl)
        n92 = Unbundle By Name(w293) -> ("Stop Condition Enable"=w282:bool, "Enable Delay (s)"=w281:dbl, "Name"=w285:string, "Threshold"=w280:dbl, "Event"=w279:i32, "num. of events"=w278:i32)
        n93 = call <instrlib>:"Config-Sampling-Parameters.vi"("VISA session"=w258, "mode (linear: 0)"=w289, "initial interval (sec)"=w288, "sampling time\n(linear/thinned-out only)"=w287, "number of samples"=w286, "error in (no error)"=w265, "sampling time limit"=w284, "num. of events"=w278, "event (val > threshold:0)"=w279, "stop condition"=w282, "hold time (sec)"=w283, "enable delay"=w281, "name"=w285, "threshold"=w280) -> ("error out"=w298:errorcluster)  [unwired: 2 in, 11 out]
        n94 = for {
          tunnel: w258 -> [w342]
          tunnel: w263 -> [w341] mode=indexing
          shift-right: [w346] -> w259
          shift-left: w298 -> [w345]
          tunnel: w264 -> [w340] mode=indexing
          tunnel: w257 -> [w337] mode=indexing
          tunnel: w256 -> [w332] mode=indexing
          shift-right: [w336] -> w254
          shift-left: w255 -> [w335]
          shift-right: [w333] -> w253
          shift-left: w255 -> [w334]
          n95 = Unbundle By Name(w341) -> ("Mode"=w338:u32, "Function"=w339:bool, "Source"=w344:dbl, "Compliance"=w343:dbl)
          n96 = case shown="True" w339 {
            tunnel: [w349 w362] -> w346
            tunnel: w345 -> [w349 w361]
            tunnel: w344 -> [_ w360]
            tunnel: w343 -> [_ w359]
            tunnel: w342 -> [_ w358]
            tunnel: w340 -> [_ w357]
            tunnel: w338 -> [_ w356]
            tunnel: w337 -> [_ w355]
            tunnel: [w348 w354] -> w336
            tunnel: w335 -> [w348 w353]
            tunnel: w334 -> [w347 w352]
            tunnel: [w347 w351] -> w333
            tunnel: w332 -> [_ w350]
            frame False {
              # "Disabled"
            }
            frame True {
              n97 = case shown="2" w356 {
                tunnel: [w363 w369] -> w362
                tunnel: w361 -> [w363 w368]
                tunnel: w360 -> [_ w367]
                tunnel: w359 -> [_ w366]
                tunnel: w358 -> [_ w365]
                tunnel: w357 -> [_ w364]
                frame 2 {
                  # "Common"
                }
                frame Default {
                  n98 = call <instrlib>:"Config-Sampling-Const-Source.vi"("compliance (SMUs only)"=w366, "error in (no error)"=w368, "source (V or A)"=w367, "unit (SMU1:0)"=w364, "VISA session"=w365) -> ("error out"=w369:errorcluster)  [unwired: 6 out]
                }
              }
              n99 = Build Array (concatenate)(w352, w350) -> (w351:string[])
              n100 = Build Array (concatenate)(w353, w355) -> (w354:string[])
            }
          }
        }
        n101 = Insert Into Array(array=w254, new element=w253) -> (w252:string[])  [unwired: 1 in]
        n102 = call <instrlib>:"Config-Display-List.vi"("error in (no error)"=w259, "list (max 8 elements)"=w252, "VISA session"=w258) -> ("error out"=w260:errorcluster)  [unwired: 1 in, 7 out]
        n103 = call <instrlib>:"Sys-Error Query.vi"("error in (no error)"=w260, "VISA session"=w258) -> ("error out"=w291:errorcluster, "messages"=w290:string)  [unwired: 1 in, 7 out]
        n104 = Unbundle By Name(w294) -> ("Status"=w295:refnum<notifier>)
        n105 = Not A Number/Path/Refnum?(number/path/refnum=w295) -> (NaN/Path/Refnum?=w296:bool)
        n106 = case shown="False" w296 {
          tunnel: w291 -> [w383 w384]
          tunnel: [w382 w384] -> w249
          tunnel: w295 -> [w381 _]
          frame False {
            n107 = Send Notification(notification="Sampling Configured", notifier=w381, error in (no error)=w383) -> (error out=w382:errorcluster)  [unwired: 1 out]
          }
          frame True {
          }
        }
        n108 = case shown="No Error" w249 {
          selector: w249 -> [w307 w311]
          tunnel: [w306 w310] -> w247
          tunnel: w248 -> [w302 w312]
          frame No Error {
            n109 = control-ref of="Instrument Status"() -> (w305:refnum<vi>)
            n110 = Unbundle By Name(w302) -> ("Instrument Status"=w303:refnum<vi>)
            n111 = Build Array(w303, w305) -> (w304:refnum<vi>[])
            n112 = call "Edit Status Indicator.vi"("error in (no error)"=w307, "State"=Instrument_Status_State."Idle", "Instrument Status Refnum"=w304) -> ("error out"=w306:errorcluster)  [unwired: 1 in, 7 out]
          }
          frame Error {
            n113 = control-ref of="Instrument Status"() -> (w315:refnum<vi>)
            n114 = Unbundle By Name(w312) -> ("Instrument Status"=w313:refnum<vi>)
            n115 = Build Array(w313, w315) -> (w314:refnum<vi>[])
            n116 = call "Edit Status Indicator.vi"("State"=Instrument_Status_State."Unknown", "Instrument Status Refnum"=w314) -> ("error out"=w309:errorcluster)  [unwired: 2 in, 7 out]
            n117 = Merge Errors(w309, w311) -> (w310:errorcluster)
          }
        }
      }
      frame "Configure Integration Time" {
        # "Number of Power Line Cycles"
        n118 = case shown="No Error" w389 {
          selector: w389 -> [w438 w442]
          tunnel: [w437 w441] -> w388
          tunnel: w386 -> [w433 w443]
          frame No Error {
            n119 = control-ref of="Instrument Status"() -> (w436:refnum<vi>)
            n120 = Unbundle By Name(w433) -> ("Instrument Status"=w434:refnum<vi>)
            n121 = Build Array(w434, w436) -> (w435:refnum<vi>[])
            n122 = call "Edit Status Indicator.vi"("error in (no error)"=w438, "State"=Instrument_Status_State."Configuring", "Instrument Status Refnum"=w435) -> ("error out"=w437:errorcluster)  [unwired: 1 in, 7 out]
          }
          frame Error {
            n123 = control-ref of="Instrument Status"() -> (w446:refnum<vi>)
            n124 = Unbundle By Name(w443) -> ("Instrument Status"=w444:refnum<vi>)
            n125 = Build Array(w444, w446) -> (w445:refnum<vi>[])
            n126 = call "Edit Status Indicator.vi"("State"=Instrument_Status_State."Unknown", "Instrument Status Refnum"=w445) -> ("error out"=w440:errorcluster)  [unwired: 2 in, 7 out]
            n127 = Merge Errors(w440, w442) -> (w441:errorcluster)
          }
        }
        n128 = Unbundle By Name(w405) -> ("Integration Time"=w393:u32, "Short Integration Time (s)"=w398:dbl, "Long Integration Time (s)"=w396:dbl, "Wait Time Parameter"=w399:dbl)
        n129 = Divide(x=w396, y=0.02) -> (x/y=w395:dbl)
        n130 = Round Toward -Infinity(1:w395) -> (0:w394:dbl)
        n131 = To Long Integer(number=w394) -> (32bit integer=w392:i32)
        n132 = case shown="0, Default" w393 {
          tunnel: [w449 w452] -> w400
          tunnel: w392 -> [w448 _]
          frame 1 {
            # "Long"
            n133 = case shown="Default" w448 {
              tunnel: [w450 w451] -> w449
              frame 1 {
                w450 = u32 1 items=["Short", "Medium", "Long"] ("Integration Time")
              }
              frame Default {
                w451 = u32 2 items=["Short", "Medium", "Long"] ("Integration Time")
              }
            }
          }
          frame 0, Default {
            w452 = u32 0 items=["Short", "Medium", "Long"] ("Integration Time")
          }
        }
        n134 = call <instrlib>:"Config-Meas-Timing.vi"("# PLCs for long integration time"=w392, "short integration time\n(rounded to the nearest multiple of 80us)"=w398, "error in (no error)"=w388, "wait time parameter"=w399, "integration time"=w400, "VISA session"=w402) -> ("error out"=w416:errorcluster)  [unwired: 5 out]
        n135 = call <instrlib>:"Misc-Query Integration-Time.vi"("VISA resource name"=w402, "error in (no error)"=w416) -> ("medium integration time"=w412:dbl, "short integration time"=w414:dbl, "long integration time"=w413:dbl, "error out"=w404:errorcluster)  [unwired: 10 out]
        n136 = Bundle By Name(cluster=T17 {"Short Integration Time"=0.00192, "Medium Integration Time"=0.02, "Long Integration Time"=0.32} ("Integration Time 2"), "Short Integration Time"=w414, "Medium Integration Time"=w412, "Long Integration Time"=w413) -> (w409:T17)
        n137 = Unbundle By Name(w386) -> ("HP Integration Time"=w410:refnum<vi>)
        n138 = Not A Number/Path/Refnum?(number/path/refnum=w410) -> (NaN/Path/Refnum?=w411:bool)
        n139 = call <instrlib>:"Sys-Error Query.vi"("error in (no error)"=w404, "VISA session"=w402) -> ("error out"=w403:errorcluster, "messages"=w401:string)  [unwired: 1 in, 7 out]
        n140 = Unbundle By Name(w406) -> ("Status"=w408:refnum<notifier>)
        n141 = case shown="False" w411 {
          tunnel: w409 -> [w459 _]
          tunnel: w410 -> [w458 _]
          frame False {
            n142 = property class="Clust (strict)"(reference=w458, "Value"=w459) -> ()  [unwired: 1 in, 2 out]
          }
          frame True {
          }
        }
        n143 = Not A Number/Path/Refnum?(number/path/refnum=w408) -> (NaN/Path/Refnum?=w407:bool)
        n144 = case shown="False" w407 {
          tunnel: w403 -> [w456 w457]
          tunnel: [w455 w457] -> w387
          tunnel: w408 -> [w454 _]
          frame False {
            n145 = Send Notification(notification="Integration Time Configured", notifier=w454, error in (no error)=w456) -> (error out=w455:errorcluster)  [unwired: 1 out]
          }
          frame True {
          }
        }
        n146 = case shown="No Error" w387 {
          selector: w387 -> [w423 w427]
          tunnel: [w422 w426] -> w385
          tunnel: w386 -> [w418 w428]
          frame No Error {
            n147 = control-ref of="Instrument Status"() -> (w421:refnum<vi>)
            n148 = Unbundle By Name(w418) -> ("Instrument Status"=w419:refnum<vi>)
            n149 = Build Array(w419, w421) -> (w420:refnum<vi>[])
            n150 = call "Edit Status Indicator.vi"("error in (no error)"=w423, "State"=Instrument_Status_State."Idle", "Instrument Status Refnum"=w420) -> ("error out"=w422:errorcluster)  [unwired: 1 in, 7 out]
          }
          frame Error {
            n151 = control-ref of="Instrument Status"() -> (w431:refnum<vi>)
            n152 = Unbundle By Name(w428) -> ("Instrument Status"=w429:refnum<vi>)
            n153 = Build Array(w429, w431) -> (w430:refnum<vi>[])
            n154 = call "Edit Status Indicator.vi"("State"=Instrument_Status_State."Unknown", "Instrument Status Refnum"=w430) -> ("error out"=w425:errorcluster)  [unwired: 2 in, 7 out]
            n155 = Merge Errors(w425, w427) -> (w426:errorcluster)
          }
        }
      }
      frame "Measure" {
        w504 = 1 items=["stop  ", "single  ", "single-append  ", "stress start  ", "continuous  ", "standby on  ", "standby off  ", "zero  "] ("function (stop:0)")
        # "Communicate Measurement"
        # "Measure"
        n156 = Unbundle By Name(w509) -> ("Instrument Status"=w475:refnum<vi>, "Status"=w508:refnum<vi>)
        n157 = call <instrlib>:"Op-Start-Stop.vi"("error in (no error)"=w510, "function (stop:0)"=w504, "wait until finish"=FALSE, "VISA resource name"=w491) -> ("error out"=w513:errorcluster)  [unwired: 1 in, 6 out]
        n158 = Unbundle By Name(w501) -> ("Status"=w500:refnum<notifier>)
        n159 = while {
          tunnel: w491 -> [w708]
          tunnel: w513 -> [w710]
          tunnel: [w697] -> w503
          tunnel: w508 -> [w701]
          tunnel: w500 -> [w693]
          tunnel: w475 -> [w695]
          stop <- w706 continue-if-true
          # "Wait for HP4155C Idle  State"
          n160 = call <instrlib>:"Misc-Query Instrument State.vi"("VISA resource name"=w708, "error in (no error)"=w710) -> ("state (unknown:0)"=w699:u16, "error out"=w691:errorcluster)  [unwired: 12 out]
          "Status" <- w699
          n161 = Not A Number/Path/Refnum?(number/path/refnum=w701) -> (NaN/Path/Refnum?=w700:bool)
          n162 = Unbundle By Name(w691) -> ("code"=w702:i32)
          n163 = control-ref of="Instrument Status"() -> (w696:refnum<vi>)
          n164 = case shown="3, 4" w699 {
            tunnel: [Instrument_Status_State."Unknown" ("State") Instrument_Status_State."Idle" ("State") Instrument_Status_State."Standby" ("State") Instrument_Status_State."Measuring" ("State")] -> w694
            frame 0, Default {
            }
            frame 1 {
            }
            frame 2 {
            }
            frame 3, 4 {
            }
          }
          n165 = case shown="2" w699 {
            tunnel: ["Unknown" "Idle" "Standby" "Measuring" "Stress Force"] -> w692
            frame 0, Default {
            }
            frame 1 {
            }
            frame 2 {
            }
            frame 3 {
            }
            frame 4 {
            }
          }
          n166 = case shown="False" w700 {
            tunnel: w701 -> [w721 _]
            tunnel: w699 -> [w720 _]
            frame False {
              n167 = property class="Enum (strict)"(reference=w721, "Value"=w720) -> ()  [unwired: 1 in, 2 out]
            }
            frame True {
            }
          }
          n168 = Not Equal?(x=w699, y=u16 1) -> (x != y?=w707:bool)
          n169 = Equal?(x=w702, y=0) -> (x = y?=w705:bool)
          n170 = Wait Until Next ms Multiple(millisecond multiple="Status Polling Time (ms)") -> ()  [unwired: 1 out]
          n171 = And(x=w705, y=w707) -> (x .and. y?=w706:bool)
          n172 = Build Array(w695, w696) -> (w698:refnum<vi>[])
          n173 = call "Edit Status Indicator.vi"("error in (no error)"=w691, "State"=w694, "Instrument Status Refnum"=w698) -> ("error out"=w697:errorcluster)  [unwired: 1 in, 7 out]
          n174 = call "Notify.vi"("String"=w692, "Notifier in"=w693) -> ()  [unwired: 9 in, 1 out]
        }
        n175 = call <instrlib>:"Sys-Error Query.vi"("error in (no error)"=w503, "VISA session"=w491) -> ("error out"=w489:errorcluster, "messages"=w502:string)  [unwired: 1 in, 7 out]
        n176 = Build Array("V1" ("V name (max 6 chars)"), "V2" ("V name (max 6 chars)"), "V3" ("V name (max 6 chars)"), "V4" ("V name (max 6 chars)")) -> (w487:string[])
        n177 = Build Array("I1" ("I name (max 6 chars)"), "I2" ("I name (max 6 chars)"), "I3" ("I name (max 6 chars)"), "I4" ("I name (max 6 chars)")) -> (w486:string[])
        n178 = case shown="\"Sampling Mode\"" w465 {
          tunnel: [w529 w615] -> w478
          tunnel: [w528 w614] -> w479
          tunnel: [w527 w613] -> w480
          tunnel: [w526 w612] -> w481
          tunnel: w491 -> [w525 w611]
          tunnel: ["@TIME" "@INDEX"] -> w490
          tunnel: w489 -> [w523 w609]
          tunnel: [w522 w608] -> w488
          tunnel: [w521 w607] -> w482
          tunnel: [w520 w606] -> w483
          tunnel: [w519 w605] -> w484
          tunnel: [w518 w604] -> w485
          tunnel: w487 -> [w516 w602]
          tunnel: w486 -> [w515 w601]
          tunnel: w477 -> [w514 _]
          tunnel: w476 -> [_ w600]
          frame "Sampling Mode" {
            w517 = dbl[] [] ("Sequence")
            n179 = for {
              shift-right: [w554] -> w529
              shift-left: w517 -> [w550]
              shift-right: [w553] -> w528
              shift-left: w517 -> [w549]
              shift-right: [w552] -> w527
              shift-left: w517 -> [w548]
              shift-right: [w551] -> w526
              shift-left: w517 -> [w547]
              tunnel: w525 -> [w546]
              shift-right: [w543] -> w521
              shift-left: w517 -> [w544]
              shift-right: [w542] -> w520
              shift-left: w517 -> [w541]
              shift-right: [w539] -> w519
              shift-left: w517 -> [w540]
              shift-right: [w537] -> w518
              shift-left: w517 -> [w538]
              shift-right: [w536] -> w522
              shift-left: w523 -> [w545]
              tunnel: w517 -> [w535]
              tunnel: w516 -> [w534] mode=indexing
              tunnel: w515 -> [w533] mode=indexing
              tunnel: w514 -> [w531] mode=indexing
              i -> [w556]
              n180 = Unbundle By Name(w531) -> ("Function"=w530:bool)
              n181 = case shown="True" w530 {
                tunnel: [w589 w599] -> w555
                tunnel: w546 -> [_ w598]
                tunnel: w545 -> [w590 w597]
                tunnel: [w590 w595] -> w536
                tunnel: w535 -> [w589 _]
                tunnel: w534 -> [_ w594]
                tunnel: w533 -> [_ w592]
                tunnel: [w589 w591] -> w532
                frame False {
                  # "SMU Inactive"
                }
                frame True {
                  # "SMU Active"
                  n182 = call <instrlib>:"Op-Download Trace.vi"("error in (no error)"=w597, "trace (variable) name"=w594, "VISA session"=w598) -> ("error out"=w596:errorcluster, "trace"=w599:dbl[], "VISA resource name out"=w593:refnum<visa-resource-name>)  [unwired: 6 out]
                  n183 = call <instrlib>:"Op-Download Trace.vi"("error in (no error)"=w596, "trace (variable) name"=w592, "VISA session"=w593) -> ("error out"=w595:errorcluster, "trace"=w591:dbl[])  [unwired: 7 out]
                }
              }
              n184 = case shown="3" w556 {
                tunnel: w555 -> [w564 w572 w580 w588]
                tunnel: [w564 w571 w579 w587] -> w554
                tunnel: [w563 w572 w578 w586] -> w553
                tunnel: [w562 w570 w580 w585] -> w552
                tunnel: [w561 w569 w577 w588] -> w551
                tunnel: w550 -> [_ w571 w579 w587]
                tunnel: w549 -> [w563 _ w578 w586]
                tunnel: w548 -> [w562 w570 _ w585]
                tunnel: w547 -> [w561 w569 w577 _]
                tunnel: [w560 w568 w575 w584] -> w543
                tunnel: w544 -> [_ w568 w575 w584]
                tunnel: [w559 w567 w574 w583] -> w542
                tunnel: w541 -> [w559 _ w574 w583]
                tunnel: w540 -> [w558 w566 _ w582]
                tunnel: [w558 w566 w576 w582] -> w539
                tunnel: w538 -> [w557 w565 w573 _]
                tunnel: [w557 w565 w573 w581] -> w537
                tunnel: w532 -> [w560 w567 w576 w581]
                frame 0, Default {
                }
                frame 1 {
                }
                frame 2 {
                }
                frame 3 {
                }
              }
            }
          }
          frame "Sweeping Mode" {
            w603 = dbl[] [] ("Sequence")
            n185 = for {
              shift-right: [w640] -> w615
              shift-left: w603 -> [w636]
              shift-right: [w639] -> w614
              shift-left: w603 -> [w635]
              shift-right: [w638] -> w613
              shift-left: w603 -> [w634]
              shift-right: [w637] -> w612
              shift-left: w603 -> [w633]
              tunnel: w611 -> [w632]
              shift-right: [w629] -> w607
              shift-left: w603 -> [w630]
              shift-right: [w628] -> w606
              shift-left: w603 -> [w627]
              shift-right: [w625] -> w605
              shift-left: w603 -> [w626]
              shift-right: [w623] -> w604
              shift-left: w603 -> [w624]
              shift-right: [w622] -> w608
              shift-left: w609 -> [w631]
              tunnel: w603 -> [w621]
              tunnel: w602 -> [w620] mode=indexing
              tunnel: w601 -> [w619] mode=indexing
              tunnel: w600 -> [w617] mode=indexing
              i -> [w642]
              n186 = Unbundle By Name(w617) -> ("Function"=w616:i32)
              n187 = case shown="Default" w616 {
                tunnel: [w675 w685] -> w641
                tunnel: w632 -> [_ w684]
                tunnel: w631 -> [w676 w683]
                tunnel: [w676 w681] -> w622
                tunnel: w621 -> [w675 _]
                tunnel: w620 -> [_ w680]
                tunnel: w619 -> [_ w678]
                tunnel: [w675 w677] -> w618
                frame 0 {
                  # "SMU Inactive"
                }
                frame Default {
                  n188 = call <instrlib>:"Op-Download Trace.vi"("error in (no error)"=w683, "trace (variable) name"=w680, "VISA session"=w684) -> ("error out"=w682:errorcluster, "trace"=w685:dbl[], "VISA resource name out"=w679:refnum<visa-resource-name>)  [unwired: 6 out]
                  n189 = call <instrlib>:"Op-Download Trace.vi"("error in (no error)"=w682, "trace (variable) name"=w678, "VISA session"=w679) -> ("error out"=w681:errorcluster, "trace"=w677:dbl[])  [unwired: 7 out]
                }
              }
              n190 = case shown="3" w642 {
                tunnel: w641 -> [w650 w658 w666 w674]
                tunnel: [w650 w657 w665 w673] -> w640
                tunnel: [w649 w658 w664 w672] -> w639
                tunnel: [w648 w656 w666 w671] -> w638
                tunnel: [w647 w655 w663 w674] -> w637
                tunnel: w636 -> [_ w657 w665 w673]
                tunnel: w635 -> [w649 _ w664 w672]
                tunnel: w634 -> [w648 w656 _ w671]
                tunnel: w633 -> [w647 w655 w663 _]
                tunnel: [w646 w654 w661 w670] -> w629
                tunnel: w630 -> [_ w654 w661 w670]
                tunnel: [w645 w653 w660 w669] -> w628
                tunnel: w627 -> [w645 _ w660 w669]
                tunnel: w626 -> [w644 w652 _ w668]
                tunnel: [w644 w652 w662 w668] -> w625
                tunnel: w624 -> [w643 w651 w659 _]
                tunnel: [w643 w651 w659 w667] -> w623
                tunnel: w618 -> [w646 w653 w662 w667]
                frame 0, Default {
                }
                frame 1 {
                }
                frame 2 {
                }
                frame 3 {
                }
              }
            }
          }
        }
        n191 = call "Parameter Analyzer Time-IDX_Download.vi"("Error In (no error)"=w488, "Trace (variable) name"=w490, "VISA session"=w491) -> ("Error Out"=w468:errorcluster, "Trace"=w511:dbl[])
        n192 = Bundle(cluster=T15 {"Sequence"=[], "V1"=[], "V2"=[], "V3"=[], "V4"=[], "I1"=[], "I2"=[], "I3"=[], "I4"=[]} ("Electrical Measurement 2"), "Sequence"=w511, "V1"=w478, "V2"=w479, "V3"=w480, "V4"=w481, "I1"=w482, "I2"=w483, "I3"=w484, "I4"=w485) -> (w470:T15)
        "Electrical Measurement" <- w470
        n193 = Unbundle By Name(w509) -> ("Plots"=w469:T6)
        n194 = Unbundle By Name(w501) -> ("Status"=w460:refnum<notifier>, "Measurement"=w506:refnum<notifier>)
        n195 = Not A Number/Path/Refnum?(number/path/refnum=w506) -> (NaN/Path/Refnum?=w505:bool)
        n196 = call "Plot Electrical Data.vi"("Plot Refnums"=w469, "Electrical Measurement"=w470, "Measurement Mode"=w465, "error in (no error)"=w468) -> ("Voltage Plot Array"=→"Voltage Plot 2":cluster{"Sequence":dbl[], "Data":dbl[]}[], "Current Plot Array"=→"Current Plot 2":cluster{"Sequence":dbl[], "Data":dbl[]}[], "Current Voltage Array"=→"Current Voltage Characteristic":cluster{"Voltage":dbl[], "Current":dbl[]}[], "Differential Resistance Array"=→"Differential Resistance":cluster{"Voltage":dbl[], "Resistance":dbl[]}[], "error out"=w466:errorcluster)  [unwired: 3 in, 4 out]
        n197 = case shown="False" w505 {
          tunnel: w468 -> [w689 w690]
          tunnel: [w688 w690] -> w463
          tunnel: w506 -> [w687 _]
          tunnel: w470 -> [w686 _]
          frame False {
            n198 = Send Notification(notification=w686, notifier=w687, error in (no error)=w689) -> (error out=w688:errorcluster)  [unwired: 1 out]
          }
          frame True {
          }
        }
        n199 = call "Notify.vi"("error in (no error)"=w463, "String"="Measurement Performed", "Notifier in"=w460) -> ("error out"=w461:errorcluster)  [unwired: 8 in]
        n200 = Merge Errors(w461, w466) -> (w467:errorcluster)
      }
      frame "Error Check" {
        n201 = call <instrlib>:"Sys-Error Query.vi"("error in (no error)"=w730, "VISA session"=w729) -> ("error out"=w731:errorcluster, "messages"=w726:string)  [unwired: 1 in, 7 out]
      }
      frame "Disconnect" {
        n202 = call <instrlib>:"Close.vi"("error in (no error)"=w746, "VISA resource name"=w745) -> ("error out"=w732:errorcluster)  [unwired: 9 out]
        n203 = case shown="No Error" w732 {
          selector: w732 -> [w752 w756]
          tunnel: [w751 w755] -> w733
          tunnel: w735 -> [w747 w757]
          frame No Error {
            n204 = control-ref of="Instrument Status"() -> (w750:refnum<vi>)
            n205 = Unbundle By Name(w747) -> ("Instrument Status"=w748:refnum<vi>)
            n206 = Build Array(w748, w750) -> (w749:refnum<vi>[])
            n207 = call "Edit Status Indicator.vi"("error in (no error)"=w752, "State"=Instrument_Status_State."Disconnected", "Instrument Status Refnum"=w749) -> ("error out"=w751:errorcluster)  [unwired: 1 in, 7 out]
          }
          frame Error {
            n208 = control-ref of="Instrument Status"() -> (w760:refnum<vi>)
            n209 = Unbundle By Name(w757) -> ("Instrument Status"=w758:refnum<vi>)
            n210 = Build Array(w758, w760) -> (w759:refnum<vi>[])
            n211 = call "Edit Status Indicator.vi"("State"=Instrument_Status_State."Unknown", "Instrument Status Refnum"=w759) -> ("error out"=w754:errorcluster)  [unwired: 2 in, 7 out]
            n212 = Merge Errors(w754, w756) -> (w755:errorcluster)
          }
        }
        n213 = Unbundle By Name(w739) -> ("Status"=w741:refnum<notifier>)
        n214 = Not A Number/Path/Refnum?(number/path/refnum=w741) -> (NaN/Path/Refnum?=w742:bool)
        n215 = case shown="False" w742 {
          tunnel: w732 -> [w765 w766]
          tunnel: [w764 w766] -> w740
          tunnel: w741 -> [w763 _]
          frame False {
            n216 = Send Notification(notification="Disconnected", notifier=w763, error in (no error)=w765) -> (error out=w764:errorcluster)  [unwired: 1 out]
          }
          frame True {
          }
        }
        n217 = Merge Errors(w740, w733) -> (w734:errorcluster)
      }
      frame "Update Refnums" {
        n218 = Unbundle By Name("Parameter Analyzer Notifiers") -> ("Status"=w770:refnum<notifier>)
        n219 = call "Notify.vi"("error in (no error)"=w768, "String"="Refnums Updated", "Notifier in"=w770) -> ("error out"=w767:errorcluster)  [unwired: 8 in]
      }
    }
  }
  "Error Messages" <- w19
  "HP Integration Time" <- w18
  "error out" <- w11
